vi "Host-Scannig-Probe-Microscope-Controller-2010-06-05-RFR-1a-version-for-MCL-drift-trial-fm-NanoH50 D082914.vi"() -> ()   [LabVIEW 2012]
uses:
  <vilib>/FPGAPlugInAG/PCI-7831R/niLvFpga_Open_PCI-7831R.vi
  <vilib>/Utility/error.llb/Error Cluster From Error Code.vi
  <vilib>/rvi/errors/niLvFpgaAdjustHostInterfaceError.vi
  <vilib>/FPGAPlugInAG/PCI-7831R/niLvFpga_Close_PCI-7831R.vi
  <vilib>/FPGAPlugInAG/PCI-7831R/niLvFpga_Run_PCI-7831R.vi
  <vilib>/Utility/file.llb/Write To Spreadsheet File (I64).vi
  <vilib>/rvi/interface/nirviOpenFPGA/nirviOpenFPGA.xnode
  Documents/FPGA-project-apporach-retraction/FPGA Bitfiles/Apporach-Retract_FPGATarget_Scannig-Probe-Mi_0gtNGMjHE5o.lvbitx
  Scannig-Probe-Microscope-Controller-2010-03-08-RFR-1a-version-for-MCL-drift-trial-fm-multiple-channels-nanoh50.vi
  <vilib>/rvi/interface/nirviMethod/nirviMethod.xnode
  <vilib>/rvi/interface/nirviReadWriteControl/nirviReadWriteControl.xnode
  <vilib>/rvi/interface/nirviCloseFPGA/nirviCloseFPGA.xnode
  <vilib>/rvi/errors/niLvFpgaMergeErrorWithErrorCode.vi
  NiFpgaLv.dll
  <vilib>/FPGAPlugInAG/PCI-7831R/niLvFpga_ReadFifo_PCI-7831R.vi
panel:
  out "fpga y images":i32
  out "hi(x)":u16[](array[numeric])=[65532, 21, 65429, 46, 65369, 15, 65513, 65465, 46, 65357, 35, 65457, 65513, 26, 65398, 44, 65387, 9, 4, 65453, 44, 65356, 26, 65480, 65489, 30, 65375, 36, 65416, 3, 18, 65446, 48, 65359, 19, 65504, 65469, 44, 65360, 34, 65444, 65519, 25, 65408, 47, 65382, 13, 65532, 65458, 44, 65353, 30, 65471, 65495, 30, 65383, 42, 65407, 6, 13, 65452, 48, 65368, 21, 65495, 65473, 39, 65364, 37, 65438, 65528, 23, 65411, 46, 65377, 13, 65524, 65460, 44, 65353, 32, 65464, 65502, 26, 65391, 43, 65397, 6, 9, 65450, 46, 65362, 25, 65486, 65480, 27, 65365, 42, 65424, 65533, 23, 65423, 47, 65371, 15, 65514, 65464, 42, 65355, 31, 65456, 65506, 26, 65394, 45, 65389, 9, 6, 65453, 47, 65354, 25, 65478, 65484, 28, 65374, 34, 65417, 0, 21, 65435, 47, 65359, 18, 65507, 65468, 46, 65356, 34, 65448, 65517, 26, 65405, 44, 65386, 11, 65535, 65457, 46, 65355, 28, 65476, 65492, 29, 65377, 42, 65410, 3, 18, 65454, 48, 65363, 20, 65501, 65473, 39, 65359, 36, 65438, 65524, 24, 65410, 46, 65380, 13, 65531, 65460, 46, 65355, 31, 65467, 65497, 28, 65384, 42, 65402, 7, 13, 65449, 46, 65368, 23, 65490, 65477, 35, 65366, 40, 65432, 65529, 22, 65417, 47, 65374, 14, 65519, 65464, 42, 65354, 31, 65460, 65501, 28, 65393, 46, 65395, 9, 8, 65453, 48, 65356, 26, 65483, 65482, 21, 65368, 39, 65423, 65533, 23, 65429, 48, 65367, 17, 65510, 65466, 46, 65357, 33, 65451, 65510, 23, 65400, 43, 65389, 10, 2, 65455, 47, 65353, 26, 65476, 65490, 28, 65378, 35, 65413]
  out "Y line":i32=81
  out "Time per step (us) /X axis sub pixels":u32=1220
  in  "X axis pixels":u16=512
  in  "Lines per second":dbl=0.2 min=1e-05 max=50.0
  in  "Time per step/ Y axis sub pixels (usec)":u32=1200
  in  "X Size (um)":dbl=10.0
  in  "X Total Range (um)":dbl=80.0
  in  "Y Size (um)":dbl=10.0
  in  "Y Total Range (um)":dbl=80.0
  in  "Y axis pixels":u16=512
  in  "Timeout FIFO":i32=-1
  in  "x initial":i16=-32760
  in  "y initial":i16=-32710
  out "X axis steps per pixel":u16=8
  in  "Number of images":u32=10000
  out "Y axis steps per pixel":u16=8
  out "Pixels for one image":i32=524288
  in  "Internal Setpoint":i16=7166
  in  "I scale":i8=-8
  in  "P scale":i8
  in  "Setpoint Control":bool=TRUE
  in  "PID gains (x 2^8)":T1={"proportional gain (Kc)"=1, "integral gain (Kc*Ts/Ti)"=11, "derivative gain (Kc*Td/Ts)"=0}
  in  "Forth/Back X axis":bool
  in  "Forth/Back Y axis":bool
  in  "Feedback loop time(uSec)":u8
  in  "Stop Feedback":bool=TRUE
  in  "Scanning On/Off":bool
  in  "control for drift correction":u32=512000
  out "Steps Per Feedback region":u16=642
  in  "Number of Feedback Regions":u32=102
  in  "upper limit regions":i16=99
  out "line shift":i32=-1
  out "line in matrix":i32=80
  out "Y Output Value":i16=-32054
  out "image indicator":i32
  out "Bottom Sensor Magnitude Image":i16[][](graph)
  out "Trace Bottom Sensor Magnitude":i16[][](graph)=[[41, 50, 79, 100, 124, 92, 130, 194, 155, 119, 90, 52, 169, 196, 52, 81, 107, 97, 38, 169, 150, 28, 89, 84, 18, 25, 51, 184, 150, 110, 155, 167, 122, 228, 203, 75, 201, 101, 167, 149, 80, 89, 32, 120, 164, 110, 260, 104, 77, 34, 69, 125, 141, 131, 177, 43, 257, 242, 80, 65, 98, 218, 145, 115, 125, 34, 174, 80, 78, 182, 63, 67, -5, 186, 59, 112, 169, 133, 153, 205, 220, 231, 179, -6, 137, 135, 104, 121, 121, 4, 32, 127, 149, 22, 158, 160, 147, 32, -108, 132, 241, 134, 185, 77, 233, 197, 268, 26, 211, 313, 123, 22, 29, 158, 139, 153, 155, 139, 230, 147, 12, 119, 36, 53, 226, 114, 18, 89, 167, 226, 89, 114, 39, 114, 146, 82, 117, 210, 120, 130, 89, 242, 66, 50, 63, 89, 215, 93, 202, 62, 217, 101, 72, 108, 107, 230, 75, 124, 178, 145, 151, 112, 161, 160, 128, 42, 134, 109, -52, 159, 142, 126, 57, 230, 7, 151, 27, 129, 87, 148, 174, 142, 215, 110, 88, 45, 88, 43, 146, 227, 61, 262, 158, 118, 154, 142, 53, 207, 196, 101, 8, 132, 58, 74, 95, 69, 131, 226, 161, 109, 62, 212, 3, 20, 207, 111, 193, 73, 242, 114, -14, 170, 48, 4, 172, 90, 96, 287, -18, 98, 30, 147, 228, 145, 109, 136, 208, 182, 156, 163, 119, 305, 172, 81, 230, 199, 73, 148, 62, 266, 63, 82, 17, 132, 77, 305, 38, 6, 50, 233, -5, 164, 215, 85, 188, 159, 89, 148, 139, 127, 68, 84, 64, 238, 9, 122, 235, 77, 234, 71, 177, 104, 123, 214, 172, 130, 85, 121, 161, 251, 152, 66, 171, 109, 58, 62, 176, 92, 94, 126, 180, 228, 42, 122, 190, 41, 40, 153, 163, 53, 217, 123, 118, 264, 64, 154, 144, 148, 118, 109, 101, 11, 203, 147, 25, 144, 81, 112, 73, 203, -57, 181, 123, 193, 104, 135, 17, 56, 129, 13, 50, 44, 147, 27, 109, 142, 56, 62, 32, 58, 140, 83, 227, 195, 134, 215, 50, 203, 102, 86, 208, 209, 139, 108, -58, 11, 72, 101, 138, 63, 137, 68, -11, 42, 1, 134, 216, 138, 188, 215, 64, 8, 187, 93, 120, 168, 70, 177, 149, 89, 212, 163, 106, 81, 168, 123, 21, 162, 185, 136, 154, 242, 215, 20, 57, 91, 132, 166, 53, 82, 128, 161, 135, 157, 35, 205, 194, 101, 103, 69, 37, 127, 227, 263, 80, 125, 186, 204, 287, 183, 120, 125, 86, 101, 166, 236, 53, 84, 129, 184, 176, 178, 174, 93, 163, 270, 115, 249, 64, 138, 89, 95, 118, 130, 80, 148, 289, 86, 28, 138, 90, -9, 254, -56, 149, 109, 109, 200, 191, 115, 157, 157, 104, 51, 114, 153, 143, 244, 163, 134, 201, 38, 224, 75, 191, 52, 102, 58, 133, 48, 107, 72, 153, 156, 112, 192, 141, 256, 86, 107, 219, 83, 42, 109, 20, 138, 149, 132, 110, 40, 88, 109], [237, 108, 67, 210, -4, 118, 207, 137, 134, 154, 46, 91, 85, 154, 186, 70, 135, 69, 110, 172, 208, 152, 193, 103, 111, 178, 97, 183, 209, 67, 119, 163, 212, 109, 20, 163, 7, 190, 70, -17, 66, 151, 91, 93, 120, 178, 145, 129, 219, 78, 111, 87, 86, 155, 94, 93, 54, 109, 153, 159, 144, 111, 80, 104, 64, 79, 156, 141, 82, 143, -2, 71, 150, 232, 121, 3, 232, 88, 36, 47, 193, 81, 106, 144, 106, 72, 124, 213, 165, 117, 153, 159, 162, 120, 325, 90, 117, 87, 87, 133, -6, 137, 137, 167, 112, 108, 23, 81, 70, 158, 146, 83, 137, -24, 100, 138, 131, 102, 95, -69, 87, 125, 183, 60, 33, 56, 167, 231, 74, 171, 165, 206, 70, 64, 21, 211, 148, 52, 153, 198, 80, 101, 140, 147, 69, 206, 166, 42, -16, 164, 160, 116, 64, 72, 121, 99, 128, 140, 85, 82, 170, 265, 192, 175, -2, 181, 123, 92, 101, 162, 136, 82, 246, 86, 9, 62, 126, 144, 57, 152, 167, 16, 94, 105, 137, 26, 186, -33, 135, 104, 136, 183, 150, 33, 124, 56, 87, 26, 196, 107, 136, 185, 156, 173, 4, 134, 42, 232, 81, 219, 55, 3, 133, -19, 83, 286, 83, 75, 38, 219, 116, 114, 189, 196, 119, 84, 196, 88, 111, 169, -24, 139, 173, 87, 230, 56, 182, 110, 155, 154, 113, 148, 155, 141, 61, 133, 88, 163, 144, 110, 241, 108, 112, 64, 194, -2, 89, 191, 94, -9, -30, 82, 203, 109, 142, 5, 71, 135, 185, 118, 98, 106, 40, 112, 120, 41, 124, 172, 67, 21, 123, 242, 256, 164, 121, 156, 87, 39, 174, 48, 107, 190, 31, 272, 98, 79, 133, -45, 80, 38, 143, 69, 151, 188, 149, 122, 97, 95, 112, -25, 208, 87, 197, 218, 72, 141, 9, 66, 35, 140, 51, 51, 196, 189, 150, 61, 183, 227, 139, -11, 150, 161, 5, 64, 174, 43, 230, 131, 25, 170, 96, 226, 93, 184, 69, 118, 240, 96, 215, 39, 169, 40, 252, 140, 135, 133, 284, 192, 100, 110, 99, 114, 56, 50, 83, 63, -8, 158, 66, -4, 168, 79, 233, 28, 35, 199, 110, 116, 141, 191, 77, 45, 123, 158, 17, 150, 162, 164, 84, 72, 90, 91, 88, 98, 195, 98, 178, 169, 217, 196, 27, 220, 92, 129, 165, 111, 150, 74, 93, 203, 103, 142, 132, 128, 13, 101, 143, 178, 72, -13, 185, -42, 134, 78, 157, 114, 112, 77, 59, 172, 105, 224, 79, 73, -16, 46, 116, 163, 134, 120, 123, 133, 81, -8, 214, 227, 117, 39, 225, 198, 12, 55, 93, 228, 90, 61, 106, 20, 57, 53, 144, 64, 67, 213, 8, 97, 232, 133, 119, 224, 70, 158, 228, 218, 154, 189, 141, 139, 183, 73, 70, 46, 202, 41, 236, 112, 94, 95, 47, 55, 45, 201, -8, 114, 136, 46, 21, 42, 137, 107, 47, 253, 20, 186, 118, 177, 163, 130, 105, 59, 214, 186]]
  out "TF Magnitude Image":i16[][](graph)
  out "Trace TF Magnitud":i16[][](graph)=[[-1059, -1061, -1058, -1061, -1059, -1062, -1059, -1060, -1061, -1060, -1059, -1061, -1060, -1059, -1062, -1061, -1059, -1061, -1061, -1059, -1060, -1060, -1063, -1061, -1062, -1062, -1059, -1056, -1062, -1058, -1060, -1059, -1061, -1060, -1059, -1061, -1058, -1061, -1060, -1062, -1061, -1059, -1060, -1060, -1061, -1059, -1057, -1060, -1061, -1060, -1059, -1060, -1060, -1060, -1060, -1060, -1058, -1060, -1058, -1061, -1060, -1058, -1060, -1061, -1059, -1059, -1060, -1059, -1062, -1059, -1061, -1060, -1061, -1060, -1060, -1060, -1060, -1059, -1061, -1059, -1059, -1057, -1063, -1058, -1061, -1061, -1061, -1061, -1059, -1060, -1061, -1059, -1062, -1059, -1059, -1060, -1059, -1060, -1061, -1060, -1060, -1059, -1060, -1060, -1058, -1057, -1062, -1060, -1059, -1059, -1058, -1060, -1061, -1060, -1059, -1059, -1062, -1059, -1060, -1060, -1058, -1061, -1062, -1060, -1058, -1062, -1053, -1061, -1058, -1060, -1060, -1059, -1062, -1060, -1061, -1056, -1059, -1058, -1058, -1059, -1059, -1062, -1061, -1058, -1060, -1060, -1062, -1061, -1061, -1061, -1061, -1059, -1059, -1058, -1060, -1058, -1061, -1060, -1062, -1060, -1061, -1058, -1057, -1060, -1061, -1062, -1060, -1061, -1060, -1060, -1060, -1058, -1060, -1059, -1060, -1060, -1062, -1059, -1058, -1060, -1060, -1063, -1061, -1058, -1061, -1059, -1061, -1061, -1061, -1057, -1059, -1058, -1061, -1061, -1061, -1061, -1062, -1061, -1061, -1059, -1059, -1058, -1061, -1061, -1062, -1059, -1058, -1061, -1060, -1061, -1059, -1058, -1060, -1060, -1058, -1060, -1059, -1062, -1060, -1061, -1061, -1060, -1062, -1061, -1059, -1062, -1062, -1059, -1062, -1061, -1061, -1060, -1060, -1060, -1059, -1059, -1059, -1062, -1059, -1059, -1060, -1060, -1061, -1059, -1059, -1060, -1061, -1059, -1060, -1059, -1059, -1060, -1060, -1060, -1062, -1059, -1060, -1062, -1059, -1057, -1061, -1059, -1057, -1060, -1057, -1058, -1059, -1058, -1060, -1059, -1059, -1060, -1059, -1059, -1060, -1062, -1055, -1060, -1059, -1058, -1059, -1059, -1059, -1061, -1060, -1059, -1057, -1059, -1059, -1061, -1060, -1058, -1057, -1061, -1062, -1060, -1060, -1058, -1061, -1059, -1058, -1058, -1061, -1061, -1061, -1060, -1062, -1061, -1060, -1059, -1058, -1062, -1061, -1058, -1061, -1058, -1059, -1059, -1061, -1062, -1061, -1061, -1060, -1061, -1052, -1060, -1062, -1060, -1061, -1059, -1060, -1060, -1061, -1059, -1061, -1061, -1061, -1062, -1061, -1062, -1061, -1061, -1060, -1060, -1060, -1061, -1059, -1063, -1062, -1061, -1062, -1062, -1060, -1062, -1060, -1060, -1060, -1062, -1058, -1059, -1060, -1057, -1059, -1060, -1064, -1061, -1059, -1059, -1059, -1061, -1059, -1059, -1061, -1058, -1061, -1059, -1058, -1058, -1060, -1061, -1061, -1060, -1058, -1060, -1060, -1060, -1062, -1061, -1059, -1059, -1059, -1059, -1059, -1059, -1059, -1060, -1061, -1059, -1058, -1058, -1061, -1057, -1057, -1060, -1061, -1058, -1061, -1061, -1055, -1059, -1060, -1059, -1061, -1060, -1059, -1057, -1059, -1062, -1060, -1061, -1061, -1058, -1061, -1060, -1061, -1057, -1061, -1059, -1061, -1059, -1056, -1059, -1060, -1059, -1062, -1059, -1059, -1059, -1059, -1057, -1058, -1060, -1060, -1060, -1057, -1057, -1058, -1061, -1062, -1060, -1059, -1060, -1060, -1059, -1060, -1061, -1060, -1059, -1061, -1059, -1058, -1061, -1059, -1058, -1061, -1060, -1060, -1057, -1060, -1062, -1059, -1059, -1058, -1062, -1058, -1062, -1059, -1060, -1061, -1058, -1060, -1061, -1057, -1059, -1062, -1061, -1059, -1061, -1059, -1060, -1063, -1059, -1059, -1060, -1063, -1061, -1059, -1059, -1059, -1059, -1058, -1063, -1060, -1060, -1061, -1059, -1062, -1063, -1060, -1058, -1059, -1058], [-1057, -1058, -1060, -1059, -1061, -1060, -1059, -1061, -1057, -1060, -1062, -1060, -1060, -1060, -1057, -1060, -1057, -1060, -1059, -1060, -1060, -1061, -1060, -1059, -1060, -1059, -1057, -1062, -1058, -1062, -1056, -1059, -1059, -1061, -1058, -1061, -1058, -1059, -1061, -1059, -1061, -1059, -1059, -1059, -1061, -1058, -1059, -1057, -1058, -1060, -1062, -1060, -1058, -1060, -1061, -1060, -1059, -1057, -1059, -1060, -1059, -1058, -1059, -1064, -1061, -1061, -1059, -1061, -1059, -1060, -1061, -1058, -1060, -1057, -1060, -1060, -1058, -1059, -1059, -1059, -1060, -1059, -1060, -1062, -1061, -1059, -1059, -1059, -1059, -1060, -1061, -1058, -1060, -1059, -1057, -1059, -1060, -1060, -1062, -1061, -1060, -1058, -1063, -1058, -1060, -1062, -1061, -1058, -1060, -1060, -1059, -1061, -1060, -1061, -1059, -1060, -1056, -1059, -1060, -1060, -1059, -1060, -1060, -1060, -1060, -1059, -1060, -1059, -1060, -1060, -1060, -1059, -1061, -1062, -1060, -1059, -1059, -1062, -1058, -1057, -1062, -1059, -1060, -1059, -1058, -1058, -1057, -1061, -1060, -1061, -1058, -1061, -1059, -1059, -1060, -1060, -1060, -1057, -1058, -1060, -1062, -1057, -1057, -1059, -1061, -1060, -1060, -1059, -1060, -1060, -1058, -1060, -1061, -1060, -1060, -1059, -1062, -1060, -1060, -1062, -1060, -1060, -1059, -1062, -1059, -1061, -1059, -1062, -1059, -1059, -1059, -1060, -1062, -1061, -1061, -1060, -1061, -1062, -1058, -1064, -1061, -1059, -1060, -1060, -1063, -1061, -1060, -1057, -1062, -1062, -1061, -1060, -1062, -1060, -1062, -1057, -1061, -1061, -1058, -1061, -1061, -1059, -1061, -1057, -1060, -1060, -1060, -1060, -1060, -1060, -1061, -1060, -1060, -1060, -1060, -1061, -1059, -1059, -1060, -1056, -1061, -1060, -1057, -1059, -1061, -1060, -1062, -1059, -1056, -1056, -1061, -1060, -1057, -1059, -1060, -1058, -1059, -1060, -1059, -1060, -1060, -1060, -1061, -1060, -1060, -1057, -1058, -1059, -1057, -1061, -1058, -1062, -1060, -1057, -1061, -1061, -1060, -1061, -1059, -1062, -1057, -1061, -1058, -1061, -1058, -1057, -1060, -1060, -1059, -1060, -1060, -1057, -1062, -1059, -1060, -1061, -1058, -1059, -1060, -1061, -1059, -1060, -1058, -1059, -1060, -1059, -1060, -1059, -1061, -1060, -1058, -1060, -1061, -1060, -1058, -1059, -1060, -1060, -1060, -1060, -1061, -1061, -1062, -1058, -1061, -1061, -1060, -1059, -1059, -1059, -1059, -1060, -1061, -1059, -1059, -1059, -1059, -1061, -1060, -1060, -1060, -1058, -1061, -1060, -1056, -1060, -1058, -1060, -1061, -1060, -1061, -1063, -1058, -1057, -1059, -1060, -1062, -1062, -1061, -1061, -1060, -1060, -1061, -1060, -1061, -1060, -1063, -1058, -1059, -1058, -1060, -1058, -1055, -1061, -1061, -1059, -1058, -1060, -1061, -1061, -1059, -1062, -1060, -1060, -1061, -1060, -1061, -1060, -1061, -1059, -1060, -1059, -1058, -1060, -1059, -1062, -1061, -1058, -1061, -1060, -1062, -1059, -1059, -1060, -1061, -1062, -1058, -1061, -1060, -1060, -1060, -1059, -1060, -1063, -1059, -1060, -1061, -1060, -1062, -1061, -1061, -1062, -1059, -1057, -1062, -1065, -1059, -1061, -1058, -1061, -1061, -1059, -1060, -1058, -1060, -1061, -1060, -1059, -1060, -1059, -1063, -1062, -1059, -1064, -1060, -1061, -1061, -1062, -1058, -1060, -1061, -1060, -1059, -1059, -1061, -1057, -1059, -1060, -1058, -1060, -1060, -1062, -1060, -1059, -1061, -1061, -1059, -1060, -1060, -1059, -1060, -1057, -1060, -1057, -1060, -1060, -1060, -1059, -1059, -1061, -1060, -1060, -1059, -1060, -1058, -1060, -1060, -1063, -1063, -1061, -1060, -1059, -1061, -1058, -1060, -1061, -1059, -1059, -1060, -1063, -1063, -1058, -1061, -1060, -1057, -1061, -1060, -1059, -1061, -1058, -1062, -1058]]
  out "Trace AI5 array":i16[][](array[numeric])=[[41, 50, 79, 100, 124, 92, 130, 194, 155, 119, 90, 52, 169, 196, 52, 81, 107, 97, 38, 169, 150, 28, 89, 84, 18, 25, 51, 184, 150, 110, 155, 167, 122, 228, 203, 75, 201, 101, 167, 149, 80, 89, 32, 120, 164, 110, 260, 104, 77, 34, 69, 125, 141, 131, 177, 43, 257, 242, 80, 65, 98, 218, 145, 115, 125, 34, 174, 80, 78, 182, 63, 67, -5, 186, 59, 112, 169, 133, 153, 205, 220, 231, 179, -6, 137, 135, 104, 121, 121, 4, 32, 127, 149, 22, 158, 160, 147, 32, -108, 132, 241, 134, 185, 77, 233, 197, 268, 26, 211, 313, 123, 22, 29, 158, 139, 153, 155, 139, 230, 147, 12, 119, 36, 53, 226, 114, 18, 89, 167, 226, 89, 114, 39, 114, 146, 82, 117, 210, 120, 130, 89, 242, 66, 50, 63, 89, 215, 93, 202, 62, 217, 101, 72, 108, 107, 230, 75, 124, 178, 145, 151, 112, 161, 160, 128, 42, 134, 109, -52, 159, 142, 126, 57, 230, 7, 151, 27, 129, 87, 148, 174, 142, 215, 110, 88, 45, 88, 43, 146, 227, 61, 262, 158, 118, 154, 142, 53, 207, 196, 101, 8, 132, 58, 74, 95, 69, 131, 226, 161, 109, 62, 212, 3, 20, 207, 111, 193, 73, 242, 114, -14, 170, 48, 4, 172, 90, 96, 287, -18, 98, 30, 147, 228, 145, 109, 136, 208, 182, 156, 163, 119, 305, 172, 81, 230, 199, 73, 148, 62, 266, 63, 82, 17, 132, 77, 305, 38, 6, 50, 233, -5, 164, 215, 85, 188, 159, 89, 148, 139, 127, 68, 84, 64, 238, 9, 122, 235, 77, 234, 71, 177, 104, 123, 214, 172, 130, 85, 121, 161, 251, 152, 66, 171, 109, 58, 62, 176, 92, 94, 126, 180, 228, 42, 122, 190, 41, 40, 153, 163, 53, 217, 123, 118, 264, 64, 154, 144, 148, 118, 109, 101, 11, 203, 147, 25, 144, 81, 112, 73, 203, -57, 181, 123, 193, 104, 135, 17, 56, 129, 13, 50, 44, 147, 27, 109, 142, 56, 62, 32, 58, 140, 83, 227, 195, 134, 215, 50, 203, 102, 86, 208, 209, 139, 108, -58, 11, 72, 101, 138, 63, 137, 68, -11, 42, 1, 134, 216, 138, 188, 215, 64, 8, 187, 93, 120, 168, 70, 177, 149, 89, 212, 163, 106, 81, 168, 123, 21, 162, 185, 136, 154, 242, 215, 20, 57, 91, 132, 166, 53, 82, 128, 161, 135, 157, 35, 205, 194, 101, 103, 69, 37, 127, 227, 263, 80, 125, 186, 204, 287, 183, 120, 125, 86, 101, 166, 236, 53, 84, 129, 184, 176, 178, 174, 93, 163, 270, 115, 249, 64, 138, 89, 95, 118, 130, 80, 148, 289, 86, 28, 138, 90, -9, 254, -56, 149, 109, 109, 200, 191, 115, 157, 157, 104, 51, 114, 153, 143, 244, 163, 134, 201, 38, 224, 75, 191, 52, 102, 58, 133, 48, 107, 72, 153, 156, 112, 192, 141, 256, 86, 107, 219, 83, 42, 109, 20, 138, 149, 132, 110, 40, 88, 109], [237, 108, 67, 210, -4, 118, 207, 137, 134, 154, 46, 91, 85, 154, 186, 70, 135, 69, 110, 172, 208, 152, 193, 103, 111, 178, 97, 183, 209, 67, 119, 163, 212, 109, 20, 163, 7, 190, 70, -17, 66, 151, 91, 93, 120, 178, 145, 129, 219, 78, 111, 87, 86, 155, 94, 93, 54, 109, 153, 159, 144, 111, 80, 104, 64, 79, 156, 141, 82, 143, -2, 71, 150, 232, 121, 3, 232, 88, 36, 47, 193, 81, 106, 144, 106, 72, 124, 213, 165, 117, 153, 159, 162, 120, 325, 90, 117, 87, 87, 133, -6, 137, 137, 167, 112, 108, 23, 81, 70, 158, 146, 83, 137, -24, 100, 138, 131, 102, 95, -69, 87, 125, 183, 60, 33, 56, 167, 231, 74, 171, 165, 206, 70, 64, 21, 211, 148, 52, 153, 198, 80, 101, 140, 147, 69, 206, 166, 42, -16, 164, 160, 116, 64, 72, 121, 99, 128, 140, 85, 82, 170, 265, 192, 175, -2, 181, 123, 92, 101, 162, 136, 82, 246, 86, 9, 62, 126, 144, 57, 152, 167, 16, 94, 105, 137, 26, 186, -33, 135, 104, 136, 183, 150, 33, 124, 56, 87, 26, 196, 107, 136, 185, 156, 173, 4, 134, 42, 232, 81, 219, 55, 3, 133, -19, 83, 286, 83, 75, 38, 219, 116, 114, 189, 196, 119, 84, 196, 88, 111, 169, -24, 139, 173, 87, 230, 56, 182, 110, 155, 154, 113, 148, 155, 141, 61, 133, 88, 163, 144, 110, 241, 108, 112, 64, 194, -2, 89, 191, 94, -9, -30, 82, 203, 109, 142, 5, 71, 135, 185, 118, 98, 106, 40, 112, 120, 41, 124, 172, 67, 21, 123, 242, 256, 164, 121, 156, 87, 39, 174, 48, 107, 190, 31, 272, 98, 79, 133, -45, 80, 38, 143, 69, 151, 188, 149, 122, 97, 95, 112, -25, 208, 87, 197, 218, 72, 141, 9, 66, 35, 140, 51, 51, 196, 189, 150, 61, 183, 227, 139, -11, 150, 161, 5, 64, 174, 43, 230, 131, 25, 170, 96, 226, 93, 184, 69, 118, 240, 96, 215, 39, 169, 40, 252, 140, 135, 133, 284, 192, 100, 110, 99, 114, 56, 50, 83, 63, -8, 158, 66, -4, 168, 79, 233, 28, 35, 199, 110, 116, 141, 191, 77, 45, 123, 158, 17, 150, 162, 164, 84, 72, 90, 91, 88, 98, 195, 98, 178, 169, 217, 196, 27, 220, 92, 129, 165, 111, 150, 74, 93, 203, 103, 142, 132, 128, 13, 101, 143, 178, 72, -13, 185, -42, 134, 78, 157, 114, 112, 77, 59, 172, 105, 224, 79, 73, -16, 46, 116, 163, 134, 120, 123, 133, 81, -8, 214, 227, 117, 39, 225, 198, 12, 55, 93, 228, 90, 61, 106, 20, 57, 53, 144, 64, 67, 213, 8, 97, 232, 133, 119, 224, 70, 158, 228, 218, 154, 189, 141, 139, 183, 73, 70, 46, 202, 41, 236, 112, 94, 95, 47, 55, 45, 201, -8, 114, 136, 46, 21, 42, 137, 107, 47, 253, 20, 186, 118, 177, 163, 130, 105, 59, 214, 186]]
  out "Trace AI5 temp":i16[](array[numeric])=[54, 151, 139, 139, 176, 3, 95, 63, 94, 117, 40, 198, 140, 226, 89, 129, 122, 115, 125, 198, 114, 199, 172, -33, 154, 113, 26, 61, 166, 124, 137, 48, 150, 145, 106, 30, 92, 95, -27, 280, 207, 128, 67, 20, 85, 155, 27, 159, 250, 127, 137, 135, 76, 149, 265, 148, 181, 6, -14, 177, 118, 132, 185, 76, 84, 23, 220, 166, 117, 73, 60, 94, 218, 108, 122, 76, 97, 57, 101, 133, 106, 52, 213, 117, 91, 203, 72, 19, 167, 107, 152, 237, 120, 175, 209, 12, 220, 53, 237, 121, 136, -82, 173, 57, 39, 127, 94, 149, 176, 184, 117, 40, 44, 118, 191, 125, 91, 45, -32, 227, 141, 182, 112, 95, 7, 45, 178, 201, 208, 181, 85, 109, 135, 49, 188, 187, 60, 54, 100, 116, 115, 130, 125, 189, 102, -61, 133, 159, 154, 107, 181, 239, 50, 117, 184, 67, 161, 149, 63, 177, 111, 121, 81, 101, 42, 277, 121, 98, 56, 128, 125, 196, 139, 155, 168, 197, 141, 114, 143, 97, 106, 42, 231, 85, 222, 139, 86, 118, 127, 86, -37, 62, 224, 9, 10, 132, 133, 213, 76, 73, 181, 46, 200, 77, 145, 208, 111, 82, 35, 123, 22, 72, 142, 99, 75, 217, 190, 189, 215, 221, 136, 138, 196, 57, 43, 145, 163, 147, 114, 97, 159, 246, 181, -17, 117, 156, 128, 86, 142, 232, 14, 218, 68, 178, 79, 142, 43, 152, 172, 104, 54, 95, 107, 163, 188, 88, 87, 160, 97, 101, 88, 34, 26, 171, 43, 45, 91, 36, 213, -103, 272, 152, 177, 143, 38, 124, 42, 162, 52, 47, 155, 131, 135, 52, 148, 152, 163, 103, 126, 185, 184, 232, 99, 47, 231, 96, 120, 194, 43, 82, 189, 262, 102, 83, 52, 156, 24, 126, 77, 195, 24, 119, 114, 134, 280, 259, 118, 39, 118, 115, 136, 190, 147, 129, 58, 132, 29, 127, 219, 59, 58, 87, 213, 126, 221, 65, 202, 54, 98, 279, -80, 98, 110, 108, 168, 79, 131, 132, -31, 124, 155, 62, 314, 26, 205, 111, -37, 15, 158, 83, 129, 13, 153, 198, 71, 85, -13, 63, 242, 108, 81, 144, 20, 175, 80, 46, 88, 207, 136, 43, 205, -17, 211, 206, 134, 90, 139, 61, 71, 170, 201, 39, 12, 295, 119, 160, 132, 14, 170, 19, 127, 78, 157, 141, 148, 127, 173, 11, 66, 178, 12, 180, 138, 231, 46, 214, 15, 146, -20, -11, 185, 91, 88, 15, 51, 101, -29, 63, 192, 120, 179, 66, 48, 85, 45, 214, 139, 24, 163, 196, 142, 88, 169, 192, 36, 141, 124, 121, 189, 139, 4, 57, 86, 56, 170, 104, 66, 201, 121, 79, 188, 126, 96, 168, 110, 251, 86, 82, 99, 131, 149, 105, 111, 79, 194, 153, 129, 65, 120, 226, 199, 103, 28, 197, 239, 277, 13, 222, 116, 74, 258, 59, 118, 336, 126, 140, 316, 51, 107, 86, 48, 36, 171, 133, 97, 114, 131, 151, 169, 39, 189, 135]
  out "Trace AI6  array":i16[][](array[numeric])=[[-1059, -1061, -1058, -1061, -1059, -1062, -1059, -1060, -1061, -1060, -1059, -1061, -1060, -1059, -1062, -1061, -1059, -1061, -1061, -1059, -1060, -1060, -1063, -1061, -1062, -1062, -1059, -1056, -1062, -1058, -1060, -1059, -1061, -1060, -1059, -1061, -1058, -1061, -1060, -1062, -1061, -1059, -1060, -1060, -1061, -1059, -1057, -1060, -1061, -1060, -1059, -1060, -1060, -1060, -1060, -1060, -1058, -1060, -1058, -1061, -1060, -1058, -1060, -1061, -1059, -1059, -1060, -1059, -1062, -1059, -1061, -1060, -1061, -1060, -1060, -1060, -1060, -1059, -1061, -1059, -1059, -1057, -1063, -1058, -1061, -1061, -1061, -1061, -1059, -1060, -1061, -1059, -1062, -1059, -1059, -1060, -1059, -1060, -1061, -1060, -1060, -1059, -1060, -1060, -1058, -1057, -1062, -1060, -1059, -1059, -1058, -1060, -1061, -1060, -1059, -1059, -1062, -1059, -1060, -1060, -1058, -1061, -1062, -1060, -1058, -1062, -1053, -1061, -1058, -1060, -1060, -1059, -1062, -1060, -1061, -1056, -1059, -1058, -1058, -1059, -1059, -1062, -1061, -1058, -1060, -1060, -1062, -1061, -1061, -1061, -1061, -1059, -1059, -1058, -1060, -1058, -1061, -1060, -1062, -1060, -1061, -1058, -1057, -1060, -1061, -1062, -1060, -1061, -1060, -1060, -1060, -1058, -1060, -1059, -1060, -1060, -1062, -1059, -1058, -1060, -1060, -1063, -1061, -1058, -1061, -1059, -1061, -1061, -1061, -1057, -1059, -1058, -1061, -1061, -1061, -1061, -1062, -1061, -1061, -1059, -1059, -1058, -1061, -1061, -1062, -1059, -1058, -1061, -1060, -1061, -1059, -1058, -1060, -1060, -1058, -1060, -1059, -1062, -1060, -1061, -1061, -1060, -1062, -1061, -1059, -1062, -1062, -1059, -1062, -1061, -1061, -1060, -1060, -1060, -1059, -1059, -1059, -1062, -1059, -1059, -1060, -1060, -1061, -1059, -1059, -1060, -1061, -1059, -1060, -1059, -1059, -1060, -1060, -1060, -1062, -1059, -1060, -1062, -1059, -1057, -1061, -1059, -1057, -1060, -1057, -1058, -1059, -1058, -1060, -1059, -1059, -1060, -1059, -1059, -1060, -1062, -1055, -1060, -1059, -1058, -1059, -1059, -1059, -1061, -1060, -1059, -1057, -1059, -1059, -1061, -1060, -1058, -1057, -1061, -1062, -1060, -1060, -1058, -1061, -1059, -1058, -1058, -1061, -1061, -1061, -1060, -1062, -1061, -1060, -1059, -1058, -1062, -1061, -1058, -1061, -1058, -1059, -1059, -1061, -1062, -1061, -1061, -1060, -1061, -1052, -1060, -1062, -1060, -1061, -1059, -1060, -1060, -1061, -1059, -1061, -1061, -1061, -1062, -1061, -1062, -1061, -1061, -1060, -1060, -1060, -1061, -1059, -1063, -1062, -1061, -1062, -1062, -1060, -1062, -1060, -1060, -1060, -1062, -1058, -1059, -1060, -1057, -1059, -1060, -1064, -1061, -1059, -1059, -1059, -1061, -1059, -1059, -1061, -1058, -1061, -1059, -1058, -1058, -1060, -1061, -1061, -1060, -1058, -1060, -1060, -1060, -1062, -1061, -1059, -1059, -1059, -1059, -1059, -1059, -1059, -1060, -1061, -1059, -1058, -1058, -1061, -1057, -1057, -1060, -1061, -1058, -1061, -1061, -1055, -1059, -1060, -1059, -1061, -1060, -1059, -1057, -1059, -1062, -1060, -1061, -1061, -1058, -1061, -1060, -1061, -1057, -1061, -1059, -1061, -1059, -1056, -1059, -1060, -1059, -1062, -1059, -1059, -1059, -1059, -1057, -1058, -1060, -1060, -1060, -1057, -1057, -1058, -1061, -1062, -1060, -1059, -1060, -1060, -1059, -1060, -1061, -1060, -1059, -1061, -1059, -1058, -1061, -1059, -1058, -1061, -1060, -1060, -1057, -1060, -1062, -1059, -1059, -1058, -1062, -1058, -1062, -1059, -1060, -1061, -1058, -1060, -1061, -1057, -1059, -1062, -1061, -1059, -1061, -1059, -1060, -1063, -1059, -1059, -1060, -1063, -1061, -1059, -1059, -1059, -1059, -1058, -1063, -1060, -1060, -1061, -1059, -1062, -1063, -1060, -1058, -1059, -1058], [-1057, -1058, -1060, -1059, -1061, -1060, -1059, -1061, -1057, -1060, -1062, -1060, -1060, -1060, -1057, -1060, -1057, -1060, -1059, -1060, -1060, -1061, -1060, -1059, -1060, -1059, -1057, -1062, -1058, -1062, -1056, -1059, -1059, -1061, -1058, -1061, -1058, -1059, -1061, -1059, -1061, -1059, -1059, -1059, -1061, -1058, -1059, -1057, -1058, -1060, -1062, -1060, -1058, -1060, -1061, -1060, -1059, -1057, -1059, -1060, -1059, -1058, -1059, -1064, -1061, -1061, -1059, -1061, -1059, -1060, -1061, -1058, -1060, -1057, -1060, -1060, -1058, -1059, -1059, -1059, -1060, -1059, -1060, -1062, -1061, -1059, -1059, -1059, -1059, -1060, -1061, -1058, -1060, -1059, -1057, -1059, -1060, -1060, -1062, -1061, -1060, -1058, -1063, -1058, -1060, -1062, -1061, -1058, -1060, -1060, -1059, -1061, -1060, -1061, -1059, -1060, -1056, -1059, -1060, -1060, -1059, -1060, -1060, -1060, -1060, -1059, -1060, -1059, -1060, -1060, -1060, -1059, -1061, -1062, -1060, -1059, -1059, -1062, -1058, -1057, -1062, -1059, -1060, -1059, -1058, -1058, -1057, -1061, -1060, -1061, -1058, -1061, -1059, -1059, -1060, -1060, -1060, -1057, -1058, -1060, -1062, -1057, -1057, -1059, -1061, -1060, -1060, -1059, -1060, -1060, -1058, -1060, -1061, -1060, -1060, -1059, -1062, -1060, -1060, -1062, -1060, -1060, -1059, -1062, -1059, -1061, -1059, -1062, -1059, -1059, -1059, -1060, -1062, -1061, -1061, -1060, -1061, -1062, -1058, -1064, -1061, -1059, -1060, -1060, -1063, -1061, -1060, -1057, -1062, -1062, -1061, -1060, -1062, -1060, -1062, -1057, -1061, -1061, -1058, -1061, -1061, -1059, -1061, -1057, -1060, -1060, -1060, -1060, -1060, -1060, -1061, -1060, -1060, -1060, -1060, -1061, -1059, -1059, -1060, -1056, -1061, -1060, -1057, -1059, -1061, -1060, -1062, -1059, -1056, -1056, -1061, -1060, -1057, -1059, -1060, -1058, -1059, -1060, -1059, -1060, -1060, -1060, -1061, -1060, -1060, -1057, -1058, -1059, -1057, -1061, -1058, -1062, -1060, -1057, -1061, -1061, -1060, -1061, -1059, -1062, -1057, -1061, -1058, -1061, -1058, -1057, -1060, -1060, -1059, -1060, -1060, -1057, -1062, -1059, -1060, -1061, -1058, -1059, -1060, -1061, -1059, -1060, -1058, -1059, -1060, -1059, -1060, -1059, -1061, -1060, -1058, -1060, -1061, -1060, -1058, -1059, -1060, -1060, -1060, -1060, -1061, -1061, -1062, -1058, -1061, -1061, -1060, -1059, -1059, -1059, -1059, -1060, -1061, -1059, -1059, -1059, -1059, -1061, -1060, -1060, -1060, -1058, -1061, -1060, -1056, -1060, -1058, -1060, -1061, -1060, -1061, -1063, -1058, -1057, -1059, -1060, -1062, -1062, -1061, -1061, -1060, -1060, -1061, -1060, -1061, -1060, -1063, -1058, -1059, -1058, -1060, -1058, -1055, -1061, -1061, -1059, -1058, -1060, -1061, -1061, -1059, -1062, -1060, -1060, -1061, -1060, -1061, -1060, -1061, -1059, -1060, -1059, -1058, -1060, -1059, -1062, -1061, -1058, -1061, -1060, -1062, -1059, -1059, -1060, -1061, -1062, -1058, -1061, -1060, -1060, -1060, -1059, -1060, -1063, -1059, -1060, -1061, -1060, -1062, -1061, -1061, -1062, -1059, -1057, -1062, -1065, -1059, -1061, -1058, -1061, -1061, -1059, -1060, -1058, -1060, -1061, -1060, -1059, -1060, -1059, -1063, -1062, -1059, -1064, -1060, -1061, -1061, -1062, -1058, -1060, -1061, -1060, -1059, -1059, -1061, -1057, -1059, -1060, -1058, -1060, -1060, -1062, -1060, -1059, -1061, -1061, -1059, -1060, -1060, -1059, -1060, -1057, -1060, -1057, -1060, -1060, -1060, -1059, -1059, -1061, -1060, -1060, -1059, -1060, -1058, -1060, -1060, -1063, -1063, -1061, -1060, -1059, -1061, -1058, -1060, -1061, -1059, -1059, -1060, -1063, -1063, -1058, -1061, -1060, -1057, -1061, -1060, -1059, -1061, -1058, -1062, -1058]]
  out "TraceAI6 temp":i16[](array[numeric])=[-1060, -1059, -1059, -1058, -1059, -1058, -1061, -1061, -1059, -1059, -1058, -1057, -1061, -1059, -1061, -1058, -1060, -1061, -1058, -1058, -1060, -1062, -1060, -1060, -1060, -1058, -1060, -1061, -1060, -1062, -1060, -1061, -1059, -1060, -1061, -1061, -1059, -1061, -1060, -1057, -1058, -1059, -1061, -1057, -1058, -1059, -1061, -1058, -1058, -1060, -1060, -1059, -1060, -1059, -1059, -1060, -1060, -1058, -1061, -1058, -1061, -1057, -1059, -1059, -1061, -1062, -1061, -1060, -1060, -1056, -1061, -1060, -1058, -1061, -1060, -1060, -1061, -1058, -1061, -1061, -1059, -1061, -1060, -1060, -1061, -1057, -1060, -1059, -1058, -1058, -1059, -1058, -1061, -1059, -1059, -1060, -1057, -1062, -1057, -1059, -1058, -1060, -1058, -1059, -1060, -1061, -1060, -1062, -1059, -1060, -1058, -1056, -1058, -1060, -1059, -1060, -1059, -1060, -1062, -1059, -1060, -1061, -1061, -1060, -1060, -1061, -1057, -1058, -1059, -1058, -1061, -1057, -1060, -1059, -1060, -1059, -1061, -1060, -1064, -1059, -1057, -1057, -1059, -1059, -1062, -1061, -1059, -1060, -1057, -1059, -1061, -1061, -1060, -1058, -1059, -1063, -1060, -1060, -1058, -1058, -1060, -1061, -1060, -1059, -1062, -1060, -1061, -1060, -1062, -1061, -1061, -1061, -1060, -1061, -1061, -1059, -1057, -1062, -1060, -1062, -1060, -1060, -1059, -1061, -1060, -1062, -1060, -1060, -1062, -1060, -1061, -1060, -1060, -1061, -1057, -1060, -1060, -1061, -1059, -1059, -1059, -1060, -1058, -1061, -1060, -1061, -1057, -1061, -1060, -1061, -1060, -1061, -1061, -1063, -1060, -1061, -1059, -1058, -1060, -1063, -1063, -1060, -1060, -1060, -1055, -1062, -1062, -1060, -1061, -1059, -1058, -1059, -1061, -1060, -1060, -1059, -1058, -1061, -1061, -1055, -1058, -1059, -1061, -1058, -1060, -1060, -1061, -1061, -1060, -1061, -1061, -1061, -1060, -1061, -1059, -1061, -1059, -1060, -1060, -1061, -1059, -1059, -1060, -1057, -1059, -1060, -1059, -1059, -1060, -1060, -1058, -1060, -1059, -1054, -1064, -1061, -1060, -1061, -1060, -1061, -1060, -1058, -1063, -1061, -1058, -1059, -1059, -1062, -1059, -1059, -1062, -1060, -1060, -1058, -1059, -1058, -1058, -1062, -1062, -1060, -1059, -1061, -1060, -1060, -1060, -1061, -1060, -1057, -1058, -1060, -1060, -1060, -1061, -1060, -1061, -1060, -1060, -1059, -1061, -1059, -1063, -1062, -1060, -1060, -1062, -1057, -1058, -1061, -1058, -1059, -1059, -1060, -1059, -1062, -1060, -1061, -1058, -1059, -1061, -1062, -1062, -1060, -1060, -1059, -1061, -1060, -1060, -1059, -1059, -1060, -1059, -1058, -1058, -1060, -1059, -1059, -1062, -1061, -1062, -1062, -1059, -1060, -1061, -1058, -1060, -1060, -1064, -1059, -1061, -1063, -1060, -1059, -1057, -1059, -1063, -1062, -1060, -1060, -1057, -1061, -1059, -1060, -1059, -1060, -1059, -1058, -1062, -1063, -1058, -1058, -1061, -1062, -1060, -1059, -1059, -1061, -1059, -1061, -1064, -1062, -1060, -1057, -1060, -1061, -1057, -1060, -1063, -1061, -1061, -1059, -1058, -1059, -1061, -1055, -1059, -1059, -1061, -1060, -1060, -1063, -1058, -1061, -1059, -1060, -1060, -1059, -1063, -1062, -1060, -1059, -1062, -1060, -1061, -1060, -1061, -1060, -1060, -1062, -1059, -1059, -1060, -1059, -1060, -1058, -1057, -1060, -1060, -1060, -1060, -1061, -1058, -1061, -1061, -1060, -1061, -1059, -1061, -1058, -1059, -1060, -1059, -1061, -1059, -1060, -1059, -1061, -1060, -1060, -1063, -1058, -1060, -1062, -1059, -1060, -1060, -1060, -1062, -1063, -1059, -1061, -1057, -1062, -1063, -1060, -1062, -1060, -1062, -1058, -1059, -1062, -1060, -1059, -1058, -1061, -1058, -1057, -1059, -1061, -1062, -1060, -1060, -1058, -1060, -1059, -1059, -1061, -1059, -1061, -1061, -1065, -1060, -1060]
  out "AI5 Back":i16[][](array[numeric])
  out "AI5 Array":i16[][](array[numeric])
  out "AI6 Array Back":i16[][](array[numeric])
  out "AI6 Array":i16[][](array[numeric])
  out "Internal Setpoint indicator":i16=7166
  out "iterations x":i32=83967
  out "Trace AI2 array":i16[][](array[numeric])=[[45, -178, 33, -89, -19, 26, -131, 45, -151, 10, 0, -80, 44, -182, 29, -62, -45, 30, -156, 41, -125, 2, 16, -83, 46, -175, 18, -40, -65, 39, -175, 36, -95, -12, 23, -123, 47, -156, 14, -10, -75, 47, -182, 30, -70, -36, 27, -149, 43, -136, 5, 12, -87, 48, -172, 23, -48, -58, 32, -170, 42, -107, -6, 23, -113, 48, -164, 14, -20, -71, 42, -181, 30, -79, -29, 25, -143, 45, -145, 8, 6, -84, 46, -182, 26, -57, -52, 25, -162, 34, -116, 1, 22, -104, 48, -174, 17, -30, -69, 45, -178, 33, -87, -21, 25, -133, 45, -151, 10, 0, -80, 46, -182, 27, -62, -42, 28, -156, 41, -125, 4, 16, -82, 49, -174, 23, -32, -64, 39, -175, 35, -99, -12, 23, -126, 45, -156, 14, -9, -76, 47, -181, 31, -69, -39, 26, -149, 43, -139, 8, 13, -85, 49, -169, 23, -46, -57, 30, -172, 42, -108, -6, 21, -118, 46, -165, 15, -19, -72, 43, -181, 32, -79, -29, 25, -143, 43, -145, 9, 7, -81, 47, -180, 29, -54, -53, 25, -164, 35, -116, -3, 23, -105, 49, -174, 18, -29, -69, 47, -177, 36, -86, -23, 26, -130, 44, -150, 10, 0, -77, 46, -179, 29, -60, -44, 30, -158, 38, -127, 3, 18, -82, 49, -175, 22, -32, -64, 42, -173, 37, -96, -13, 25, -127, 47, -156, 13, -8, -75, 46, -181, 33, -68, -37, 28, -150, 41, -136, 5, 12, -88, 48, -171, 24, -47, -55, 32, -171, 41, -107, -7, 24, -119, 45, -165, 16, -18, -74, 43, -182, 31, -79, -30, 28, -139, 43, -146, 8, 6, -83, 46, -179, 27, -52, -49, 27, -162, 34, -118, -1, 21, -102, 45, -174, 18, -31, -69, 47, -176, 36, -86, -20, 27, -132, 46, -152, 9, -1, -79, 48, -180, 27, -62, -42, 29, -155, 39, -126, 4, 16, -83, 48, -174, 22, -35, -65, 43, -173, 37, -96, -12, 23, -124, 46, -160, 12, -7, -74, 44, -181, 32, -67, -37, 29, -146, 42, -136, 4, 12, -87, 47, -172, 24, -46, -56, 31, -168, 42, -106, -6, 22, -113, 48, -164, 14, -20, -71, 43, -178, 31, -78, -28, 28, -140, 44, -143, 9, 7, -83, 48, -181, 27, -56, -50, 27, -163, 35, -116, 0, 20, -104, 47, -174, 19, -30, -67, 46, -176, 33, -87, -18, 27, -130, 46, -150, 11, 0, -78, 46, -182, 27, -63, -42, 30, -158, 42, -127, 3, 16, -81, 49, -174, 19, -41, -65, 40, -173, 35, -99, -12, 25, -126, 45, -159, 12, -9, -76, 46, -183, 33, -72, -36, 27, -149, 42, -137, 5, 13, -86, 48, -171, 23, -51, -57, 28, -169, 41, -108, -5, 24, -114, 48, -165, 17, -21, -73, 42, -180, 31, -78, -30, 26, -142, 43, -145, 9, 5, -81, 49, -178, 25, -57, -51, 27, -164, 36, -120, 0, 19, -100, 49, -175, 18, -32, -71, 45, -178, 32, -89, -19, 26, -129, 47, -149, 12, -2, -79, 47, -180, 27, -62, -44], [-82, 32, -177, 42, -72, -22, 15, -169, 47, -110, 22, -6, -112, 42, -169, 27, -55, -49, -62, 28, -182, 45, -77, 0, 10, -153, 46, -133, 26, -22, -87, 36, -177, 47, -66, -30, 17, -173, 46, -103, 19, -1, -118, 34, -165, 26, -51, -53, 25, -179, 46, -81, 6, 9, -146, 43, -140, 24, -29, -80, 32, -181, 43, -71, -21, 17, -165, 46, -115, 24, -5, -108, 39, -168, 30, -56, -48, 23, -174, 47, -87, 12, 6, -138, 42, -149, 28, -37, -70, 32, -180, 45, -73, -9, 15, -160, 46, -126, 24, -13, -98, 40, -174, 40, -65, -39, 21, -170, 48, -82, 16, 3, -128, 40, -158, 30, -43, -62, 29, -179, 46, -77, 1, 12, -151, 44, -129, 24, -18, -90, 34, -177, 47, -67, -30, 18, -174, 46, -100, 21, 1, -118, 34, -162, 24, -51, -56, 27, -179, 49, -81, 6, 8, -146, 42, -141, 26, -28, -80, 33, -181, 40, -73, -20, 16, -165, 48, -117, 23, -8, -110, 42, -172, 27, -57, -49, 22, -173, 48, -86, 13, 7, -137, 43, -146, 27, -39, -71, 29, -182, 46, -75, -10, 12, -157, 45, -126, 24, -11, -100, 34, -174, 39, -63, -44, 20, -170, 50, -80, 17, 6, -131, 42, -159, 27, -43, -65, 27, -181, 45, -79, -2, 9, -153, 46, -128, 23, -18, -88, 34, -177, 45, -68, -31, 17, -176, 50, -99, 22, 1, -118, 35, -161, 29, -50, -54, 27, -182, 47, -84, 6, 9, -146, 44, -140, 26, -29, -80, 33, -179, 42, -71, -23, 18, -163, 47, -111, 23, -3, -110, 42, -168, 29, -55, -49, 22, -175, 46, -87, 12, 6, -137, 44, -149, 27, -35, -69, 31, -183, 44, -75, -11, 13, -161, 46, -123, 25, -12, -98, 38, -172, 39, -63, -40, 21, -174, 48, -84, 17, 5, -130, 40, -154, 29, -44, -64, 28, -182, 45, -79, 0, 10, -153, 46, -129, 27, -17, -87, 34, -175, 46, -68, -31, 19, -175, 47, -101, 21, 1, -117, 36, -161, 28, -48, -55, 26, -181, 47, -83, 5, 8, -148, 45, -140, 26, -26, -78, 32, -176, 43, -71, -22, 17, -168, 47, -110, 24, -5, -109, 41, -169, 26, -54, -49, 25, -173, 48, -85, 10, 4, -137, 42, -146, 27, -32, -69, 32, -180, 45, -74, -10, 13, -160, 45, -128, 22, -12, -100, 38, -172, 42, -62, -41, 21, -170, 48, -81, 16, 5, -131, 41, -155, 29, -41, -64, 29, -181, 48, -77, -1, 10, -152, 45, -132, 24, -19, -90, 36, -175, 45, -67, -30, 20, -176, 48, -99, 18, 1, -119, 36, -161, 27, -51, -56, 27, -180, 48, -81, 6, 9, -147, 43, -139, 24, -28, -81, 33, -179, 43, -71, -23, 16, -166, 46, -108, 22, -4, -111, 41, -168, 27, -57, -50, 25, -174, 49, -86, 9, 4, -137, 44, -147, 26, -36, -72, 32, -181, 47, -75, -10, 14, -160, 46, -125, 23, -10, -99, 39, -174, 39, -64, -41, 22, -171, 49, -81, 16, 3, -128, 43, -158, 31]]
  out "TraceAI2 array temp":i16[](array[numeric])=[-26, 25, -140, 43, -150, 7, 3, -83, 46, -180, 28, -55, -49, 28, -163, 35, -121, 1, 19, -98, 48, -178, 19, -33, -69, 46, -178, 35, -90, -17, 24, -128, 44, -157, 9, -4, -79, 46, -182, 30, -63, -41, 30, -155, 41, -130, 3, 14, -83, 49, -169, 23, -45, -63, 40, -173, 39, -99, -10, 24, -126, 44, -164, 13, -13, -77, 44, -181, 32, -72, -33, 28, -144, 43, -137, 5, 9, -88, 47, -178, 22, -52, -55, 27, -168, 42, -111, -5, 23, -109, 48, -166, 15, -23, -71, 43, -182, 31, -82, -30, 25, -139, 44, -149, 10, 4, -81, 47, -182, 28, -58, -51, 29, -161, 36, -118, 2, 19, -95, 47, -178, 17, -34, -69, 47, -177, 33, -90, -19, 25, -131, 47, -154, 11, -2, -79, 45, -184, 28, -63, -42, 29, -155, 43, -131, 6, 17, -80, 47, -170, 19, -43, -65, 39, -175, 38, -99, -10, 23, -123, 47, -162, 14, -10, -75, 46, -182, 31, -72, -35, 27, -149, 43, -140, 5, 11, -85, 46, -174, 21, -50, -58, 27, -170, 41, -110, -4, 23, -113, 49, -165, 16, -20, -72, 43, -182, 31, -78, -30, 25, -140, 44, -147, 9, 4, -80, 47, -181, 26, -55, -50, 28, -161, 35, -118, 1, 20, -100, 49, -175, 18, -30, -69, 44, -178, 34, -88, -21, 26, -132, 45, -152, 11, -2, -77, 48, -182, 30, -62, -43, 29, -157, 41, -128, 4, 17, -81, 50, -172, 22, -38, -62, 40, -174, 37, -98, -13, 23, -122, 46, -158, 13, -10, -75, 47, -182, 33, -71, -37, 27, -148, 41, -136, 7, 13, -84, 48, -172, 24, -46, -56, 31, -170, 40, -107, -7, 24, -116, 47, -165, 16, -18, -72, 43, -181, 34, -79, -30, 26, -141, 43, -145, 9, 7, -82, 47, -178, 26, -55, -51, 27, -165, 35, -117, 1, 21, -101, 47, -174, 19, -29, -67, 46, -178, 35, -85, -22, 24, -134, 44, -151, 11, 0, -80, 46, -180, 28, -62, -45, 29, -159, 40, -126, 3, 16, -83, 48, -175, 22, -37, -64, 40, -175, 35, -97, -13, 25, -127, 46, -158, 13, -8, -77, 47, -179, 33, -67, -37, 26, -152, 44, -137, 5, 13, -86, 48, -172, 23, -46, -57, 36, -171, 40, -108, -7, 22, -122, 45, -168, 15, -18, -73, 45, -183, 31, -74, -32, 26, -143, 43, -146, 8, 8, -85, 48, -179, 26, -51, -51, 24, -164, 36, -115, -3, 20, -107, 47, -173, 19, -27, -69, 46, -177, 35, -86, -23, 26, -135, 41, -152, 8, 0, -80, 45, -180, 27, -60, -44, 31, -158, 38, -123, 1, 18, -86, 48, -177, 19, -36, -66, 42, -176, 35, -92, -16, 24, -126, 48, -158, 11, -5, -78, 48, -181, 30, -67, -40, 30, -151, 42, -132, 4, 13, -86, 46, -169, 22, -46, -60, 39, -170, 41, -102, -9, 23, -126, 47, -165, 13, -15, -73, 42, -181, 31, -73, -34, 30, -144, 43, -141, 7, 8, -87, 47, -181, 24, -51, -56, 27, -167, 41, -111]
  out "Trace Topography Array":i32[][](array[numeric])=[[2578410, 2578426, 2578418, 2578413, 2578392, 2578366, 2578366, 2578368, 2578377, 2578391, 2578393, 2578372, 2578349, 2578326, 2578333, 2578351, 2578378, 2578397, 2578411, 2578417, 2578388, 2578381, 2578388, 2578373, 2578375, 2578370, 2578352, 2578351, 2578349, 2578349, 2578329, 2578325, 2578341, 2578362, 2578357, 2578378, 2578397, 2578402, 2578414, 2578425, 2578437, 2578433, 2578422, 2578434, 2578407, 2578414, 2578430, 2578435, 2578443, 2578426, 2578435, 2578433, 2578438, 2578465, 2578492, 2578523, 2578533, 2578536, 2578545, 2578550, 2578565, 2578583, 2578580, 2578579, 2578566, 2578544, 2578562, 2578565, 2578572, 2578582, 2578597, 2578618, 2578638, 2578657, 2578673, 2578683, 2578690, 2578698, 2578703, 2578712, 2578717, 2578698, 2578699, 2578665, 2578667, 2578658, 2578648, 2578649, 2578647, 2578657, 2578677, 2578696, 2578724, 2578728, 2578751, 2578768, 2578763, 2578775, 2578766, 2578759, 2578740, 2578730, 2578721, 2578706, 2578697, 2578700, 2578690, 2578698, 2578720, 2578756, 2578789, 2578820, 2578841, 2578862, 2578864, 2578874, 2578873, 2578860, 2578848, 2578842, 2578831, 2578816, 2578809, 2578805, 2578792, 2578810, 2578816, 2578829, 2578835, 2578849, 2578857, 2578876, 2578897, 2578902, 2578900, 2578883, 2578874, 2578870, 2578834, 2578846, 2578835, 2578828, 2578827, 2578831, 2578846, 2578850, 2578877, 2578915, 2578931, 2578946, 2578962, 2578968, 2578971, 2578983, 2578991, 2578992, 2578978, 2578977, 2578989, 2578989, 2578998, 2579005, 2579001, 2579015, 2579038, 2579045, 2579071, 2579105, 2579131, 2579147, 2579175, 2579192, 2579208, 2579225, 2579238, 2579251, 2579258, 2579279, 2579290, 2579297, 2579301, 2579302, 2579308, 2579314, 2579324, 2579326, 2579329, 2579347, 2579375, 2579402, 2579418, 2579429, 2579443, 2579444, 2579450, 2579455, 2579465, 2579471, 2579491, 2579482, 2579492, 2579488, 2579502, 2579499, 2579515, 2579530, 2579544, 2579549, 2579534, 2579526, 2579526, 2579522, 2579545, 2579568, 2579564, 2579575, 2579577, 2579579, 2579597, 2579618, 2579650, 2579664, 2579654, 2579657, 2579668, 2579654, 2579678, 2579682, 2579677, 2579694, 2579690, 2579699, 2579706, 2579718, 2579727, 2579724, 2579747, 2579761, 2579796, 2579808, 2579832, 2579856, 2579848, 2579848, 2579835, 2579829, 2579835, 2579830, 2579830, 2579846, 2579864, 2579861, 2579869, 2579887, 2579908, 2579921, 2579930, 2579953, 2579969, 2579992, 2580010, 2580008, 2580022, 2580019, 2580020, 2580003, 2580015, 2580029, 2580023, 2580034, 2580054, 2580053, 2580054, 2580058, 2580074, 2580090, 2580115, 2580122, 2580131, 2580130, 2580151, 2580158, 2580161, 2580166, 2580163, 2580161, 2580170, 2580186, 2580198, 2580217, 2580219, 2580227, 2580251, 2580281, 2580286, 2580303, 2580310, 2580295, 2580289, 2580299, 2580294, 2580300, 2580305, 2580304, 2580312, 2580310, 2580309, 2580323, 2580346, 2580363, 2580395, 2580394, 2580403, 2580398, 2580419, 2580429, 2580447, 2580469, 2580471, 2580479, 2580494, 2580491, 2580506, 2580516, 2580508, 2580510, 2580513, 2580500, 2580520, 2580526, 2580555, 2580560, 2580568, 2580600, 2580602, 2580614, 2580613, 2580607, 2580609, 2580605, 2580607, 2580621, 2580608, 2580614, 2580618, 2580613, 2580637, 2580672, 2580683, 2580696, 2580710, 2580742, 2580750, 2580767, 2580789, 2580792, 2580809, 2580836, 2580822, 2580820, 2580823, 2580825, 2580825, 2580826, 2580821, 2580815, 2580837, 2580847, 2580852, 2580839, 2580852, 2580861, 2580879, 2580895, 2580915, 2580946, 2580960, 2580982, 2580991, 2580993, 2581001, 2581003, 2581005, 2581008, 2581024, 2581036, 2581036, 2581038, 2581029, 2581013, 2581017, 2581035, 2581057, 2581081, 2581103, 2581111, 2581118, 2581123, 2581130, 2581162, 2581186, 2581204, 2581198, 2581201, 2581200, 2581203, 2581243, 2581267, 2581284, 2581288, 2581268, 2581256, 2581248, 2581248, 2581252, 2581271, 2581281, 2581295, 2581280, 2581297, 2581312, 2581331, 2581346, 2581358, 2581373, 2581394, 2581410, 2581410, 2581413, 2581440, 2581456, 2581439, 2581449, 2581465, 2581464, 2581474, 2581469, 2581476, 2581489, 2581502, 2581513, 2581517, 2581532, 2581534, 2581538, 2581538, 2581547, 2581553, 2581554, 2581566, 2581577, 2581577, 2581582, 2581601, 2581617, 2581635, 2581639, 2581631, 2581632, 2581636, 2581643, 2581670, 2581686, 2581687, 2581695, 2581695, 2581706, 2581714, 2581736, 2581749, 2581748, 2581750, 2581767, 2581774, 2581769, 2581774, 2581775, 2581781, 2581767, 2581781, 2581797, 2581827, 2581838, 2581837, 2581859, 2581862, 2581861, 2581858, 2581883, 2581900, 2581918, 2581917, 2581928, 2581964, 2581976, 2582013, 2582004, 2582004, 2581998, 2581967, 2581970, 2581978, 2581980, 2581986, 2581999, 2581994, 2581987, 2581992, 2582001, 2582011, 2582026, 2582035], [2578296, 2578308, 2578305, 2578316, 2578335, 2578347, 2578370, 2578369, 2578388, 2578405, 2578431, 2578437, 2578452, 2578453, 2578460, 2578460, 2578464, 2578457, 2578470, 2578490, 2578495, 2578510, 2578506, 2578505, 2578515, 2578519, 2578522, 2578518, 2578542, 2578565, 2578576, 2578601, 2578619, 2578616, 2578619, 2578637, 2578652, 2578656, 2578632, 2578634, 2578629, 2578619, 2578631, 2578637, 2578641, 2578630, 2578619, 2578625, 2578635, 2578669, 2578688, 2578694, 2578705, 2578707, 2578722, 2578736, 2578744, 2578751, 2578737, 2578742, 2578746, 2578747, 2578752, 2578772, 2578785, 2578786, 2578780, 2578783, 2578788, 2578782, 2578795, 2578813, 2578815, 2578839, 2578839, 2578835, 2578838, 2578859, 2578874, 2578893, 2578912, 2578921, 2578930, 2578939, 2578936, 2578943, 2578966, 2579002, 2579023, 2579033, 2579051, 2579059, 2579052, 2579050, 2579069, 2579070, 2579077, 2579087, 2579091, 2579101, 2579093, 2579113, 2579120, 2579126, 2579137, 2579149, 2579157, 2579164, 2579175, 2579185, 2579182, 2579162, 2579155, 2579132, 2579145, 2579158, 2579148, 2579154, 2579154, 2579162, 2579155, 2579148, 2579156, 2579175, 2579178, 2579202, 2579216, 2579217, 2579223, 2579234, 2579241, 2579258, 2579266, 2579275, 2579255, 2579263, 2579267, 2579277, 2579289, 2579312, 2579319, 2579329, 2579321, 2579332, 2579330, 2579330, 2579337, 2579345, 2579367, 2579372, 2579355, 2579367, 2579379, 2579386, 2579388, 2579382, 2579391, 2579400, 2579391, 2579388, 2579382, 2579386, 2579387, 2579403, 2579419, 2579422, 2579433, 2579422, 2579435, 2579469, 2579492, 2579511, 2579549, 2579578, 2579577, 2579597, 2579618, 2579641, 2579655, 2579675, 2579700, 2579717, 2579740, 2579760, 2579778, 2579796, 2579813, 2579813, 2579814, 2579833, 2579856, 2579878, 2579891, 2579891, 2579891, 2579881, 2579882, 2579890, 2579889, 2579896, 2579901, 2579922, 2579935, 2579933, 2579957, 2579965, 2579977, 2579989, 2579993, 2580012, 2580009, 2580017, 2580022, 2580034, 2580035, 2580036, 2580032, 2580042, 2580060, 2580072, 2580084, 2580090, 2580110, 2580117, 2580136, 2580128, 2580132, 2580151, 2580155, 2580169, 2580149, 2580149, 2580146, 2580148, 2580151, 2580151, 2580153, 2580159, 2580185, 2580190, 2580184, 2580191, 2580205, 2580221, 2580250, 2580262, 2580271, 2580278, 2580298, 2580298, 2580308, 2580317, 2580322, 2580349, 2580352, 2580373, 2580384, 2580392, 2580393, 2580392, 2580407, 2580423, 2580418, 2580413, 2580418, 2580411, 2580419, 2580413, 2580412, 2580419, 2580422, 2580439, 2580436, 2580447, 2580467, 2580480, 2580489, 2580503, 2580517, 2580534, 2580545, 2580561, 2580570, 2580563, 2580570, 2580580, 2580577, 2580591, 2580588, 2580583, 2580602, 2580608, 2580606, 2580620, 2580612, 2580618, 2580624, 2580644, 2580674, 2580675, 2580699, 2580705, 2580707, 2580715, 2580726, 2580722, 2580719, 2580716, 2580725, 2580725, 2580753, 2580771, 2580776, 2580773, 2580780, 2580794, 2580792, 2580802, 2580816, 2580816, 2580816, 2580842, 2580858, 2580865, 2580879, 2580883, 2580899, 2580907, 2580900, 2580905, 2580919, 2580922, 2580936, 2580939, 2580962, 2580980, 2581011, 2581018, 2581015, 2581021, 2581036, 2581049, 2581058, 2581069, 2581072, 2581069, 2581064, 2581075, 2581068, 2581068, 2581089, 2581086, 2581105, 2581112, 2581118, 2581137, 2581155, 2581174, 2581197, 2581209, 2581211, 2581230, 2581248, 2581254, 2581273, 2581267, 2581254, 2581242, 2581240, 2581248, 2581253, 2581274, 2581272, 2581265, 2581276, 2581272, 2581284, 2581291, 2581304, 2581331, 2581341, 2581347, 2581342, 2581335, 2581336, 2581347, 2581351, 2581356, 2581363, 2581380, 2581384, 2581404, 2581429, 2581439, 2581469, 2581482, 2581483, 2581486, 2581478, 2581477, 2581456, 2581443, 2581434, 2581422, 2581429, 2581426, 2581434, 2581446, 2581449, 2581449, 2581492, 2581511, 2581525, 2581550, 2581566, 2581570, 2581578, 2581591, 2581604, 2581600, 2581595, 2581606, 2581615, 2581618, 2581613, 2581608, 2581626, 2581622, 2581629, 2581654, 2581686, 2581714, 2581736, 2581761, 2581764, 2581759, 2581760, 2581760, 2581755, 2581769, 2581771, 2581756, 2581755, 2581751, 2581759, 2581755, 2581750, 2581757, 2581753, 2581758, 2581779, 2581804, 2581820, 2581846, 2581850, 2581846, 2581845, 2581849, 2581836, 2581834, 2581830, 2581814, 2581845, 2581859, 2581872, 2581895, 2581894, 2581902, 2581916, 2581939, 2581949, 2581966, 2581976, 2581997, 2582004, 2582021, 2582021, 2582019, 2582019, 2582011, 2581998, 2582005, 2581989, 2581990, 2581994, 2581994, 2582011, 2581993, 2581993, 2581988, 2581985, 2581987, 2581990, 2582004, 2581993, 2582006, 2582016, 2582049, 2582067, 2582092, 2582101, 2582097, 2582091, 2582083, 2582079, 2582069, 2582071, 2582056, 2582049, 2582044, 2582033, 2582029]]
  out "Trace Topography Array temp":i32[](array[numeric])=[2578273, 2578265, 2578249, 2578244, 2578242, 2578236, 2578264, 2578277, 2578285, 2578291, 2578290, 2578284, 2578284, 2578284, 2578294, 2578294, 2578315, 2578302, 2578286, 2578284, 2578290, 2578299, 2578317, 2578333, 2578349, 2578362, 2578357, 2578366, 2578359, 2578377, 2578374, 2578365, 2578381, 2578376, 2578381, 2578390, 2578390, 2578384, 2578386, 2578383, 2578392, 2578401, 2578402, 2578406, 2578420, 2578418, 2578411, 2578418, 2578418, 2578412, 2578417, 2578429, 2578457, 2578473, 2578488, 2578484, 2578488, 2578493, 2578481, 2578481, 2578475, 2578476, 2578488, 2578491, 2578514, 2578519, 2578543, 2578556, 2578540, 2578532, 2578518, 2578513, 2578520, 2578501, 2578513, 2578517, 2578538, 2578559, 2578574, 2578593, 2578603, 2578610, 2578627, 2578622, 2578637, 2578642, 2578631, 2578634, 2578621, 2578619, 2578603, 2578592, 2578583, 2578593, 2578587, 2578588, 2578582, 2578582, 2578599, 2578609, 2578636, 2578660, 2578689, 2578704, 2578709, 2578721, 2578723, 2578724, 2578713, 2578705, 2578701, 2578705, 2578683, 2578692, 2578704, 2578722, 2578737, 2578751, 2578765, 2578765, 2578764, 2578784, 2578778, 2578775, 2578777, 2578762, 2578745, 2578746, 2578742, 2578737, 2578736, 2578740, 2578751, 2578757, 2578771, 2578787, 2578800, 2578829, 2578828, 2578848, 2578835, 2578828, 2578833, 2578829, 2578816, 2578829, 2578826, 2578838, 2578842, 2578838, 2578848, 2578846, 2578843, 2578859, 2578881, 2578902, 2578929, 2578933, 2578965, 2578987, 2578999, 2579008, 2579023, 2579021, 2579010, 2579022, 2579029, 2579014, 2579019, 2579027, 2579028, 2579056, 2579065, 2579079, 2579100, 2579122, 2579137, 2579155, 2579174, 2579214, 2579205, 2579222, 2579222, 2579204, 2579201, 2579199, 2579207, 2579211, 2579230, 2579241, 2579237, 2579240, 2579254, 2579280, 2579301, 2579328, 2579344, 2579368, 2579387, 2579388, 2579396, 2579390, 2579390, 2579382, 2579353, 2579367, 2579362, 2579372, 2579376, 2579364, 2579372, 2579390, 2579394, 2579428, 2579435, 2579458, 2579471, 2579470, 2579499, 2579496, 2579505, 2579523, 2579503, 2579500, 2579490, 2579498, 2579513, 2579511, 2579519, 2579534, 2579547, 2579576, 2579601, 2579615, 2579637, 2579639, 2579646, 2579666, 2579677, 2579693, 2579679, 2579691, 2579687, 2579678, 2579680, 2579674, 2579692, 2579698, 2579710, 2579709, 2579707, 2579712, 2579725, 2579725, 2579745, 2579753, 2579765, 2579801, 2579807, 2579803, 2579799, 2579805, 2579819, 2579826, 2579830, 2579845, 2579848, 2579834, 2579847, 2579833, 2579829, 2579827, 2579824, 2579845, 2579863, 2579879, 2579887, 2579886, 2579918, 2579932, 2579947, 2579958, 2579973, 2579958, 2579969, 2579967, 2579970, 2579988, 2579983, 2579994, 2579986, 2579993, 2580022, 2580036, 2580038, 2580063, 2580076, 2580084, 2580091, 2580103, 2580128, 2580136, 2580150, 2580143, 2580144, 2580147, 2580148, 2580166, 2580150, 2580151, 2580160, 2580166, 2580164, 2580186, 2580197, 2580210, 2580219, 2580234, 2580240, 2580244, 2580268, 2580282, 2580302, 2580304, 2580295, 2580281, 2580286, 2580307, 2580322, 2580341, 2580354, 2580347, 2580351, 2580360, 2580366, 2580383, 2580395, 2580393, 2580400, 2580398, 2580400, 2580405, 2580399, 2580413, 2580402, 2580408, 2580409, 2580400, 2580401, 2580420, 2580431, 2580442, 2580460, 2580467, 2580483, 2580492, 2580498, 2580503, 2580497, 2580512, 2580504, 2580497, 2580506, 2580511, 2580504, 2580503, 2580510, 2580524, 2580531, 2580535, 2580545, 2580546, 2580565, 2580580, 2580586, 2580607, 2580613, 2580611, 2580621, 2580647, 2580663, 2580669, 2580674, 2580689, 2580662, 2580655, 2580657, 2580654, 2580654, 2580664, 2580675, 2580674, 2580665, 2580694, 2580713, 2580730, 2580762, 2580774, 2580801, 2580830, 2580835, 2580842, 2580837, 2580842, 2580842, 2580837, 2580844, 2580843, 2580834, 2580843, 2580834, 2580858, 2580862, 2580880, 2580901, 2580904, 2580916, 2580925, 2580944, 2580964, 2580969, 2580978, 2581002, 2580996, 2580990, 2580988, 2581003, 2581020, 2581028, 2581037, 2581060, 2581061, 2581064, 2581082, 2581071, 2581082, 2581079, 2581076, 2581068, 2581068, 2581066, 2581071, 2581080, 2581096, 2581102, 2581111, 2581141, 2581148, 2581170, 2581197, 2581233, 2581240, 2581238, 2581236, 2581234, 2581217, 2581237, 2581256, 2581254, 2581265, 2581265, 2581265, 2581259, 2581258, 2581284, 2581281, 2581298, 2581308, 2581344, 2581358, 2581368, 2581383, 2581398, 2581403, 2581417, 2581405, 2581396, 2581397, 2581373, 2581376, 2581373, 2581371, 2581370, 2581372, 2581365, 2581375, 2581377, 2581387, 2581409, 2581421, 2581456, 2581474, 2581468, 2581481, 2581487, 2581503, 2581506, 2581500, 2581509, 2581515, 2581509, 2581491, 2581493, 2581491, 2581507, 2581511, 2581509, 2581513, 2581523, 2581533, 2581530, 2581535]
  out "Trace AI0 Array":i16[][](array[numeric])=[[80, -305, 87, -353, 20, 35, -176, 95, -394, 58, -111, -77, 89, -347, 82, -308, -11, 55, -233, 92, -393, 51, -27, -96, 94, -378, 71, -240, -45, 74, -282, 87, -365, 33, 25, -159, 95, -391, 61, -146, -67, 87, -335, 80, -324, -3, 51, -215, 94, -395, 51, -49, -95, 93, -363, 76, -273, -34, 62, -277, 93, -374, 38, 13, -137, 95, -389, 65, -183, -59, 82, -320, 82, -340, 9, 40, -192, 95, -401, 55, -82, -87, 91, -362, 77, -292, -24, 57, -250, 87, -385, 45, -5, -123, 96, -392, 66, -221, -53, 80, -304, 86, -356, 21, 30, -178, 94, -395, 57, -113, -78, 87, -346, 78, -308, -12, 55, -234, 89, -392, 50, -26, -96, 94, -379, 72, -236, -43, 71, -286, 87, -369, 31, 22, -160, 94, -395, 62, -149, -69, 85, -341, 82, -328, -2, 46, -213, 92, -395, 52, -56, -98, 92, -363, 76, -269, -32, 64, -272, 91, -377, 38, 15, -145, 93, -390, 63, -181, -61, 82, -321, 82, -341, 10, 41, -197, 92, -398, 56, -80, -84, 91, -358, 77, -288, -24, 53, -254, 87, -385, 45, -4, -126, 95, -390, 67, -217, -54, 82, -304, 86, -353, 20, 33, -175, 95, -397, 58, -110, -74, 89, -350, 79, -311, -13, 54, -234, 92, -391, 48, -27, -92, 91, -378, 72, -243, -43, 72, -291, 87, -366, 30, 23, -163, 96, -390, 60, -146, -68, 87, -336, 82, -324, 0, 51, -216, 92, -396, 53, -51, -95, 94, -361, 75, -272, -33, 62, -268, 90, -378, 36, 13, -143, 94, -389, 64, -181, -63, 81, -323, 86, -343, 9, 41, -197, 93, -390, 57, -80, -87, 91, -358, 79, -295, -23, 55, -252, 86, -386, 43, -9, -120, 97, -390, 67, -221, -51, 79, -304, 87, -355, 22, 33, -178, 93, -400, 59, -111, -79, 90, -348, 78, -310, -11, 55, -232, 92, -391, 46, -26, -92, 95, -375, 69, -233, -45, 73, -285, 90, -366, 32, 26, -159, 95, -395, 62, -148, -71, 85, -338, 84, -325, -2, 49, -215, 93, -398, 54, -52, -93, 93, -360, 72, -276, -33, 62, -271, 91, -378, 42, 14, -142, 96, -389, 67, -185, -62, 81, -323, 83, -339, 9, 39, -195, 93, -396, 55, -79, -87, 90, -365, 78, -294, -25, 56, -251, 86, -384, 45, -7, -117, 93, -388, 68, -216, -52, 81, -303, 84, -354, 22, 33, -172, 93, -394, 60, -118, -77, 89, -344, 80, -308, -11, 53, -231, 90, -391, 50, -29, -88, 95, -375, 70, -254, -47, 74, -281, 91, -371, 31, 25, -156, 97, -393, 63, -149, -69, 86, -331, 81, -327, 0, 49, -214, 92, -396, 55, -54, -94, 91, -361, 75, -272, -31, 59, -272, 91, -377, 42, 12, -140, 96, -388, 66, -189, -61, 83, -314, 83, -342, 11, 40, -194, 92, -397, 55, -84, -81, 92, -358, 77, -293, -20, 55, -252, 87, -387, 47, -6, -116, 96, -389, 68, -225, -52, 78, -302, 86, -356, 23, 34, -169, 95, -396, 60, -120, -76, 87, -347, 80, -310, -7], [-342, 80, -313, 82, -58, -196, 66, -389, 96, -132, 5, 45, -377, 90, -264, 59, -27, -280, -311, 76, -349, 88, -76, -113, 57, -396, 94, -175, 34, 18, -351, 85, -305, 82, -53, -219, 69, -386, 94, -123, -5, 44, -386, 86, -254, 53, -21, -292, 76, -361, 89, -83, -83, 55, -399, 95, -192, 39, 11, -342, 83, -319, 80, -54, -185, 68, -389, 93, -136, 11, 40, -377, 89, -270, 62, -31, -274, 76, -359, 92, -94, -52, 54, -396, 92, -213, 46, 3, -328, 81, -333, 85, -69, -151, 64, -393, 94, -159, 19, 31, -371, 89, -288, 71, -43, -249, 70, -370, 95, -88, -28, 51, -391, 91, -231, 55, -7, -307, 80, -347, 88, -74, -114, 60, -391, 97, -175, 35, 22, -355, 87, -302, 81, -53, -226, 68, -387, 94, -110, -6, 46, -385, 86, -249, 54, -20, -294, 77, -356, 90, -85, -84, 56, -394, 95, -191, 39, 11, -340, 83, -316, 80, -60, -187, 64, -388, 96, -138, 10, 39, -378, 91, -270, 61, -34, -270, 72, -357, 92, -92, -56, 52, -396, 92, -212, 50, 2, -327, 84, -331, 87, -69, -155, 61, -393, 95, -154, 25, 36, -367, 89, -291, 72, -42, -252, 71, -371, 93, -93, -29, 51, -393, 94, -231, 53, -10, -313, 80, -344, 88, -75, -111, 60, -394, 95, -166, 32, 23, -355, 86, -301, 79, -50, -222, 69, -388, 95, -116, -7, 46, -384, 87, -248, 56, -21, -294, 77, -357, 93, -82, -88, 58, -391, 93, -193, 40, 11, -343, 83, -316, 84, -59, -191, 67, -386, 96, -137, 11, 40, -379, 92, -269, 59, -31, -275, 73, -359, 93, -93, -53, 52, -397, 92, -212, 48, -1, -326, 82, -331, 86, -65, -152, 60, -390, 94, -158, 23, 36, -366, 90, -282, 72, -42, -250, 73, -369, 93, -92, -28, 49, -393, 91, -228, 55, -9, -312, 79, -341, 88, -75, -115, 58, -394, 93, -174, 32, 22, -352, 86, -302, 78, -49, -219, 67, -387, 93, -115, -5, 45, -386, 89, -245, 54, -16, -288, 79, -355, 91, -85, -83, 55, -397, 97, -191, 40, 12, -341, 83, -321, 81, -59, -191, 64, -387, 94, -131, 10, 40, -377, 92, -266, 59, -29, -274, 75, -360, 91, -87, -63, 51, -395, 93, -211, 47, 1, -326, 84, -331, 85, -67, -155, 62, -390, 96, -157, 21, 32, -369, 88, -285, 72, -40, -254, 70, -368, 95, -91, -29, 51, -399, 92, -231, 50, -10, -312, 79, -346, 87, -73, -119, 58, -396, 95, -172, 32, 24, -361, 86, -297, 79, -50, -227, 67, -388, 94, -117, -11, 49, -385, 87, -249, 53, -16, -295, 77, -355, 89, -78, -83, 56, -397, 94, -193, 41, 12, -344, 86, -315, 82, -63, -189, 65, -388, 95, -131, 11, 39, -379, 88, -269, 57, -28, -275, 76, -361, 90, -90, -55, 55, -393, 93, -210, 48, 3, -327, 82, -330, 86, -67, -154, 62, -392, 94, -156, 23, 35, -363, 88, -282, 72, -42, -251, 70, -372, 95, -89, -30, 50, -393, 92, -232, 55]]
  out "Trace AI0 array temp":i16[](array[numeric])=[12, 37, -191, 94, -398, 58, -90, -81, 91, -356, 77, -298, -18, 58, -246, 88, -389, 49, -11, -113, 95, -389, 69, -231, -50, 80, -299, 84, -360, 26, 30, -169, 94, -395, 59, -123, -74, 87, -342, 80, -315, -7, 49, -228, 93, -395, 49, -33, -95, 95, -368, 69, -257, -42, 70, -282, 87, -370, 36, 20, -152, 93, -391, 64, -160, -65, 85, -330, 83, -330, 5, 45, -206, 93, -395, 53, -59, -94, 92, -362, 75, -280, -27, 58, -267, 91, -375, 45, 9, -132, 96, -388, 65, -193, -59, 81, -318, 83, -347, 12, 38, -189, 94, -398, 56, -89, -81, 89, -354, 78, -295, -20, 54, -247, 87, -388, 46, -11, -112, 94, -387, 68, -224, -48, 79, -302, 85, -353, 27, 30, -170, 94, -395, 58, -117, -75, 88, -345, 77, -314, -8, 52, -231, 90, -394, 49, -32, -94, 93, -370, 73, -254, -44, 70, -285, 90, -367, 31, 19, -156, 95, -393, 62, -155, -65, 84, -329, 83, -324, -3, 45, -211, 93, -395, 53, -56, -92, 91, -364, 74, -276, -31, 59, -272, 90, -379, 41, 9, -134, 96, -391, 65, -192, -60, 82, -319, 82, -343, 16, 40, -192, 94, -398, 55, -85, -82, 92, -359, 77, -296, -20, 55, -250, 86, -385, 45, -8, -117, 95, -390, 68, -220, -53, 81, -301, 86, -354, 21, 32, -173, 95, -397, 58, -108, -80, 87, -344, 81, -316, -6, 55, -231, 94, -391, 52, -29, -92, 96, -374, 69, -249, -42, 72, -289, 88, -367, 32, 21, -156, 96, -393, 61, -149, -67, 86, -334, 80, -326, 1, 48, -212, 92, -398, 54, -49, -91, 93, -360, 75, -276, -30, 59, -274, 89, -379, 41, 11, -139, 95, -390, 67, -186, -61, 83, -323, 87, -340, 8, 40, -195, 95, -397, 56, -79, -87, 89, -357, 77, -287, -22, 57, -251, 88, -388, 49, -5, -120, 93, -389, 69, -220, -52, 80, -303, 84, -356, 21, 29, -178, 96, -399, 56, -113, -74, 89, -350, 79, -310, -10, 48, -235, 91, -391, 49, -26, -98, 94, -377, 72, -246, -45, 75, -289, 89, -367, 30, 27, -160, 94, -392, 60, -143, -69, 86, -337, 82, -320, 0, 51, -216, 92, -394, 53, -48, -95, 94, -360, 74, -269, -33, 64, -274, 92, -375, 38, 13, -146, 95, -391, 67, -174, -65, 83, -325, 82, -336, 7, 42, -198, 95, -397, 57, -75, -83, 91, -361, 76, -288, -23, 53, -258, 87, -381, 43, 4, -127, 94, -389, 67, -210, -55, 82, -307, 85, -351, 18, 34, -184, 95, -401, 57, -101, -79, 90, -351, 79, -307, -16, 57, -240, 90, -390, 49, -20, -96, 94, -384, 69, -241, -51, 75, -290, 87, -361, 29, 27, -163, 94, -391, 59, -133, -72, 88, -341, 82, -318, -6, 53, -222, 93, -391, 50, -41, -95, 93, -362, 73, -260, -40, 71, -278, 91, -374, 36, 16, -156, 94, -390, 64, -164, -62, 82, -327, 84, -330, 3, 44, -203, 94, -393, 55, -67, -94, 95, -364, 74, -280, -28, 56, -263, 88, -382]
  out "X Output Value":i16=-32760
  out "AI2 Array back":i16[][](array[numeric])
  out "AI0 back":i16[][](array[numeric])
  out "Topography Array back":i32[][](array[numeric])
  out "Command Out":i16=-32767
  out "counter":i16
  in  "Topo Prefix 2":string
  in  "Topo Prefix 1":string
  in  "Phase Prefix 2":string
  in  "Phase Prefix 1":string
  in  "Freq Prefix 2":string
  in  "Freq Prefix 1":string
  in  "Data Directory":path=path "C:/Users/Rodolfo/Documents/LAB/2013-02-24-SPM-data"
  out "Inidicator  forth/back  Y axis":i8=1
  out "Topography Image":i32[][](graph)
  out "Trace  Topography":i32[][](graph)=[[2578410, 2578426, 2578418, 2578413, 2578392, 2578366, 2578366, 2578368, 2578377, 2578391, 2578393, 2578372, 2578349, 2578326, 2578333, 2578351, 2578378, 2578397, 2578411, 2578417, 2578388, 2578381, 2578388, 2578373, 2578375, 2578370, 2578352, 2578351, 2578349, 2578349, 2578329, 2578325, 2578341, 2578362, 2578357, 2578378, 2578397, 2578402, 2578414, 2578425, 2578437, 2578433, 2578422, 2578434, 2578407, 2578414, 2578430, 2578435, 2578443, 2578426, 2578435, 2578433, 2578438, 2578465, 2578492, 2578523, 2578533, 2578536, 2578545, 2578550, 2578565, 2578583, 2578580, 2578579, 2578566, 2578544, 2578562, 2578565, 2578572, 2578582, 2578597, 2578618, 2578638, 2578657, 2578673, 2578683, 2578690, 2578698, 2578703, 2578712, 2578717, 2578698, 2578699, 2578665, 2578667, 2578658, 2578648, 2578649, 2578647, 2578657, 2578677, 2578696, 2578724, 2578728, 2578751, 2578768, 2578763, 2578775, 2578766, 2578759, 2578740, 2578730, 2578721, 2578706, 2578697, 2578700, 2578690, 2578698, 2578720, 2578756, 2578789, 2578820, 2578841, 2578862, 2578864, 2578874, 2578873, 2578860, 2578848, 2578842, 2578831, 2578816, 2578809, 2578805, 2578792, 2578810, 2578816, 2578829, 2578835, 2578849, 2578857, 2578876, 2578897, 2578902, 2578900, 2578883, 2578874, 2578870, 2578834, 2578846, 2578835, 2578828, 2578827, 2578831, 2578846, 2578850, 2578877, 2578915, 2578931, 2578946, 2578962, 2578968, 2578971, 2578983, 2578991, 2578992, 2578978, 2578977, 2578989, 2578989, 2578998, 2579005, 2579001, 2579015, 2579038, 2579045, 2579071, 2579105, 2579131, 2579147, 2579175, 2579192, 2579208, 2579225, 2579238, 2579251, 2579258, 2579279, 2579290, 2579297, 2579301, 2579302, 2579308, 2579314, 2579324, 2579326, 2579329, 2579347, 2579375, 2579402, 2579418, 2579429, 2579443, 2579444, 2579450, 2579455, 2579465, 2579471, 2579491, 2579482, 2579492, 2579488, 2579502, 2579499, 2579515, 2579530, 2579544, 2579549, 2579534, 2579526, 2579526, 2579522, 2579545, 2579568, 2579564, 2579575, 2579577, 2579579, 2579597, 2579618, 2579650, 2579664, 2579654, 2579657, 2579668, 2579654, 2579678, 2579682, 2579677, 2579694, 2579690, 2579699, 2579706, 2579718, 2579727, 2579724, 2579747, 2579761, 2579796, 2579808, 2579832, 2579856, 2579848, 2579848, 2579835, 2579829, 2579835, 2579830, 2579830, 2579846, 2579864, 2579861, 2579869, 2579887, 2579908, 2579921, 2579930, 2579953, 2579969, 2579992, 2580010, 2580008, 2580022, 2580019, 2580020, 2580003, 2580015, 2580029, 2580023, 2580034, 2580054, 2580053, 2580054, 2580058, 2580074, 2580090, 2580115, 2580122, 2580131, 2580130, 2580151, 2580158, 2580161, 2580166, 2580163, 2580161, 2580170, 2580186, 2580198, 2580217, 2580219, 2580227, 2580251, 2580281, 2580286, 2580303, 2580310, 2580295, 2580289, 2580299, 2580294, 2580300, 2580305, 2580304, 2580312, 2580310, 2580309, 2580323, 2580346, 2580363, 2580395, 2580394, 2580403, 2580398, 2580419, 2580429, 2580447, 2580469, 2580471, 2580479, 2580494, 2580491, 2580506, 2580516, 2580508, 2580510, 2580513, 2580500, 2580520, 2580526, 2580555, 2580560, 2580568, 2580600, 2580602, 2580614, 2580613, 2580607, 2580609, 2580605, 2580607, 2580621, 2580608, 2580614, 2580618, 2580613, 2580637, 2580672, 2580683, 2580696, 2580710, 2580742, 2580750, 2580767, 2580789, 2580792, 2580809, 2580836, 2580822, 2580820, 2580823, 2580825, 2580825, 2580826, 2580821, 2580815, 2580837, 2580847, 2580852, 2580839, 2580852, 2580861, 2580879, 2580895, 2580915, 2580946, 2580960, 2580982, 2580991, 2580993, 2581001, 2581003, 2581005, 2581008, 2581024, 2581036, 2581036, 2581038, 2581029, 2581013, 2581017, 2581035, 2581057, 2581081, 2581103, 2581111, 2581118, 2581123, 2581130, 2581162, 2581186, 2581204, 2581198, 2581201, 2581200, 2581203, 2581243, 2581267, 2581284, 2581288, 2581268, 2581256, 2581248, 2581248, 2581252, 2581271, 2581281, 2581295, 2581280, 2581297, 2581312, 2581331, 2581346, 2581358, 2581373, 2581394, 2581410, 2581410, 2581413, 2581440, 2581456, 2581439, 2581449, 2581465, 2581464, 2581474, 2581469, 2581476, 2581489, 2581502, 2581513, 2581517, 2581532, 2581534, 2581538, 2581538, 2581547, 2581553, 2581554, 2581566, 2581577, 2581577, 2581582, 2581601, 2581617, 2581635, 2581639, 2581631, 2581632, 2581636, 2581643, 2581670, 2581686, 2581687, 2581695, 2581695, 2581706, 2581714, 2581736, 2581749, 2581748, 2581750, 2581767, 2581774, 2581769, 2581774, 2581775, 2581781, 2581767, 2581781, 2581797, 2581827, 2581838, 2581837, 2581859, 2581862, 2581861, 2581858, 2581883, 2581900, 2581918, 2581917, 2581928, 2581964, 2581976, 2582013, 2582004, 2582004, 2581998, 2581967, 2581970, 2581978, 2581980, 2581986, 2581999, 2581994, 2581987, 2581992, 2582001, 2582011, 2582026, 2582035], [2578296, 2578308, 2578305, 2578316, 2578335, 2578347, 2578370, 2578369, 2578388, 2578405, 2578431, 2578437, 2578452, 2578453, 2578460, 2578460, 2578464, 2578457, 2578470, 2578490, 2578495, 2578510, 2578506, 2578505, 2578515, 2578519, 2578522, 2578518, 2578542, 2578565, 2578576, 2578601, 2578619, 2578616, 2578619, 2578637, 2578652, 2578656, 2578632, 2578634, 2578629, 2578619, 2578631, 2578637, 2578641, 2578630, 2578619, 2578625, 2578635, 2578669, 2578688, 2578694, 2578705, 2578707, 2578722, 2578736, 2578744, 2578751, 2578737, 2578742, 2578746, 2578747, 2578752, 2578772, 2578785, 2578786, 2578780, 2578783, 2578788, 2578782, 2578795, 2578813, 2578815, 2578839, 2578839, 2578835, 2578838, 2578859, 2578874, 2578893, 2578912, 2578921, 2578930, 2578939, 2578936, 2578943, 2578966, 2579002, 2579023, 2579033, 2579051, 2579059, 2579052, 2579050, 2579069, 2579070, 2579077, 2579087, 2579091, 2579101, 2579093, 2579113, 2579120, 2579126, 2579137, 2579149, 2579157, 2579164, 2579175, 2579185, 2579182, 2579162, 2579155, 2579132, 2579145, 2579158, 2579148, 2579154, 2579154, 2579162, 2579155, 2579148, 2579156, 2579175, 2579178, 2579202, 2579216, 2579217, 2579223, 2579234, 2579241, 2579258, 2579266, 2579275, 2579255, 2579263, 2579267, 2579277, 2579289, 2579312, 2579319, 2579329, 2579321, 2579332, 2579330, 2579330, 2579337, 2579345, 2579367, 2579372, 2579355, 2579367, 2579379, 2579386, 2579388, 2579382, 2579391, 2579400, 2579391, 2579388, 2579382, 2579386, 2579387, 2579403, 2579419, 2579422, 2579433, 2579422, 2579435, 2579469, 2579492, 2579511, 2579549, 2579578, 2579577, 2579597, 2579618, 2579641, 2579655, 2579675, 2579700, 2579717, 2579740, 2579760, 2579778, 2579796, 2579813, 2579813, 2579814, 2579833, 2579856, 2579878, 2579891, 2579891, 2579891, 2579881, 2579882, 2579890, 2579889, 2579896, 2579901, 2579922, 2579935, 2579933, 2579957, 2579965, 2579977, 2579989, 2579993, 2580012, 2580009, 2580017, 2580022, 2580034, 2580035, 2580036, 2580032, 2580042, 2580060, 2580072, 2580084, 2580090, 2580110, 2580117, 2580136, 2580128, 2580132, 2580151, 2580155, 2580169, 2580149, 2580149, 2580146, 2580148, 2580151, 2580151, 2580153, 2580159, 2580185, 2580190, 2580184, 2580191, 2580205, 2580221, 2580250, 2580262, 2580271, 2580278, 2580298, 2580298, 2580308, 2580317, 2580322, 2580349, 2580352, 2580373, 2580384, 2580392, 2580393, 2580392, 2580407, 2580423, 2580418, 2580413, 2580418, 2580411, 2580419, 2580413, 2580412, 2580419, 2580422, 2580439, 2580436, 2580447, 2580467, 2580480, 2580489, 2580503, 2580517, 2580534, 2580545, 2580561, 2580570, 2580563, 2580570, 2580580, 2580577, 2580591, 2580588, 2580583, 2580602, 2580608, 2580606, 2580620, 2580612, 2580618, 2580624, 2580644, 2580674, 2580675, 2580699, 2580705, 2580707, 2580715, 2580726, 2580722, 2580719, 2580716, 2580725, 2580725, 2580753, 2580771, 2580776, 2580773, 2580780, 2580794, 2580792, 2580802, 2580816, 2580816, 2580816, 2580842, 2580858, 2580865, 2580879, 2580883, 2580899, 2580907, 2580900, 2580905, 2580919, 2580922, 2580936, 2580939, 2580962, 2580980, 2581011, 2581018, 2581015, 2581021, 2581036, 2581049, 2581058, 2581069, 2581072, 2581069, 2581064, 2581075, 2581068, 2581068, 2581089, 2581086, 2581105, 2581112, 2581118, 2581137, 2581155, 2581174, 2581197, 2581209, 2581211, 2581230, 2581248, 2581254, 2581273, 2581267, 2581254, 2581242, 2581240, 2581248, 2581253, 2581274, 2581272, 2581265, 2581276, 2581272, 2581284, 2581291, 2581304, 2581331, 2581341, 2581347, 2581342, 2581335, 2581336, 2581347, 2581351, 2581356, 2581363, 2581380, 2581384, 2581404, 2581429, 2581439, 2581469, 2581482, 2581483, 2581486, 2581478, 2581477, 2581456, 2581443, 2581434, 2581422, 2581429, 2581426, 2581434, 2581446, 2581449, 2581449, 2581492, 2581511, 2581525, 2581550, 2581566, 2581570, 2581578, 2581591, 2581604, 2581600, 2581595, 2581606, 2581615, 2581618, 2581613, 2581608, 2581626, 2581622, 2581629, 2581654, 2581686, 2581714, 2581736, 2581761, 2581764, 2581759, 2581760, 2581760, 2581755, 2581769, 2581771, 2581756, 2581755, 2581751, 2581759, 2581755, 2581750, 2581757, 2581753, 2581758, 2581779, 2581804, 2581820, 2581846, 2581850, 2581846, 2581845, 2581849, 2581836, 2581834, 2581830, 2581814, 2581845, 2581859, 2581872, 2581895, 2581894, 2581902, 2581916, 2581939, 2581949, 2581966, 2581976, 2581997, 2582004, 2582021, 2582021, 2582019, 2582019, 2582011, 2581998, 2582005, 2581989, 2581990, 2581994, 2581994, 2582011, 2581993, 2581993, 2581988, 2581985, 2581987, 2581990, 2582004, 2581993, 2582006, 2582016, 2582049, 2582067, 2582092, 2582101, 2582097, 2582091, 2582083, 2582079, 2582069, 2582071, 2582056, 2582049, 2582044, 2582033, 2582029]]
  out "Topography Array":i32[][](array[numeric])
  in  "New Image":bool
  out "error out 2":errorcluster
  out "error out":errorcluster
  out "Bottom Sensor Phase  Image":i16[][](graph)
  out "Trace Bottom Sensor Phase":i16[][](graph)=[[80, -305, 87, -353, 20, 35, -176, 95, -394, 58, -111, -77, 89, -347, 82, -308, -11, 55, -233, 92, -393, 51, -27, -96, 94, -378, 71, -240, -45, 74, -282, 87, -365, 33, 25, -159, 95, -391, 61, -146, -67, 87, -335, 80, -324, -3, 51, -215, 94, -395, 51, -49, -95, 93, -363, 76, -273, -34, 62, -277, 93, -374, 38, 13, -137, 95, -389, 65, -183, -59, 82, -320, 82, -340, 9, 40, -192, 95, -401, 55, -82, -87, 91, -362, 77, -292, -24, 57, -250, 87, -385, 45, -5, -123, 96, -392, 66, -221, -53, 80, -304, 86, -356, 21, 30, -178, 94, -395, 57, -113, -78, 87, -346, 78, -308, -12, 55, -234, 89, -392, 50, -26, -96, 94, -379, 72, -236, -43, 71, -286, 87, -369, 31, 22, -160, 94, -395, 62, -149, -69, 85, -341, 82, -328, -2, 46, -213, 92, -395, 52, -56, -98, 92, -363, 76, -269, -32, 64, -272, 91, -377, 38, 15, -145, 93, -390, 63, -181, -61, 82, -321, 82, -341, 10, 41, -197, 92, -398, 56, -80, -84, 91, -358, 77, -288, -24, 53, -254, 87, -385, 45, -4, -126, 95, -390, 67, -217, -54, 82, -304, 86, -353, 20, 33, -175, 95, -397, 58, -110, -74, 89, -350, 79, -311, -13, 54, -234, 92, -391, 48, -27, -92, 91, -378, 72, -243, -43, 72, -291, 87, -366, 30, 23, -163, 96, -390, 60, -146, -68, 87, -336, 82, -324, 0, 51, -216, 92, -396, 53, -51, -95, 94, -361, 75, -272, -33, 62, -268, 90, -378, 36, 13, -143, 94, -389, 64, -181, -63, 81, -323, 86, -343, 9, 41, -197, 93, -390, 57, -80, -87, 91, -358, 79, -295, -23, 55, -252, 86, -386, 43, -9, -120, 97, -390, 67, -221, -51, 79, -304, 87, -355, 22, 33, -178, 93, -400, 59, -111, -79, 90, -348, 78, -310, -11, 55, -232, 92, -391, 46, -26, -92, 95, -375, 69, -233, -45, 73, -285, 90, -366, 32, 26, -159, 95, -395, 62, -148, -71, 85, -338, 84, -325, -2, 49, -215, 93, -398, 54, -52, -93, 93, -360, 72, -276, -33, 62, -271, 91, -378, 42, 14, -142, 96, -389, 67, -185, -62, 81, -323, 83, -339, 9, 39, -195, 93, -396, 55, -79, -87, 90, -365, 78, -294, -25, 56, -251, 86, -384, 45, -7, -117, 93, -388, 68, -216, -52, 81, -303, 84, -354, 22, 33, -172, 93, -394, 60, -118, -77, 89, -344, 80, -308, -11, 53, -231, 90, -391, 50, -29, -88, 95, -375, 70, -254, -47, 74, -281, 91, -371, 31, 25, -156, 97, -393, 63, -149, -69, 86, -331, 81, -327, 0, 49, -214, 92, -396, 55, -54, -94, 91, -361, 75, -272, -31, 59, -272, 91, -377, 42, 12, -140, 96, -388, 66, -189, -61, 83, -314, 83, -342, 11, 40, -194, 92, -397, 55, -84, -81, 92, -358, 77, -293, -20, 55, -252, 87, -387, 47, -6, -116, 96, -389, 68, -225, -52, 78, -302, 86, -356, 23, 34, -169, 95, -396, 60, -120, -76, 87, -347, 80, -310, -7], [-342, 80, -313, 82, -58, -196, 66, -389, 96, -132, 5, 45, -377, 90, -264, 59, -27, -280, -311, 76, -349, 88, -76, -113, 57, -396, 94, -175, 34, 18, -351, 85, -305, 82, -53, -219, 69, -386, 94, -123, -5, 44, -386, 86, -254, 53, -21, -292, 76, -361, 89, -83, -83, 55, -399, 95, -192, 39, 11, -342, 83, -319, 80, -54, -185, 68, -389, 93, -136, 11, 40, -377, 89, -270, 62, -31, -274, 76, -359, 92, -94, -52, 54, -396, 92, -213, 46, 3, -328, 81, -333, 85, -69, -151, 64, -393, 94, -159, 19, 31, -371, 89, -288, 71, -43, -249, 70, -370, 95, -88, -28, 51, -391, 91, -231, 55, -7, -307, 80, -347, 88, -74, -114, 60, -391, 97, -175, 35, 22, -355, 87, -302, 81, -53, -226, 68, -387, 94, -110, -6, 46, -385, 86, -249, 54, -20, -294, 77, -356, 90, -85, -84, 56, -394, 95, -191, 39, 11, -340, 83, -316, 80, -60, -187, 64, -388, 96, -138, 10, 39, -378, 91, -270, 61, -34, -270, 72, -357, 92, -92, -56, 52, -396, 92, -212, 50, 2, -327, 84, -331, 87, -69, -155, 61, -393, 95, -154, 25, 36, -367, 89, -291, 72, -42, -252, 71, -371, 93, -93, -29, 51, -393, 94, -231, 53, -10, -313, 80, -344, 88, -75, -111, 60, -394, 95, -166, 32, 23, -355, 86, -301, 79, -50, -222, 69, -388, 95, -116, -7, 46, -384, 87, -248, 56, -21, -294, 77, -357, 93, -82, -88, 58, -391, 93, -193, 40, 11, -343, 83, -316, 84, -59, -191, 67, -386, 96, -137, 11, 40, -379, 92, -269, 59, -31, -275, 73, -359, 93, -93, -53, 52, -397, 92, -212, 48, -1, -326, 82, -331, 86, -65, -152, 60, -390, 94, -158, 23, 36, -366, 90, -282, 72, -42, -250, 73, -369, 93, -92, -28, 49, -393, 91, -228, 55, -9, -312, 79, -341, 88, -75, -115, 58, -394, 93, -174, 32, 22, -352, 86, -302, 78, -49, -219, 67, -387, 93, -115, -5, 45, -386, 89, -245, 54, -16, -288, 79, -355, 91, -85, -83, 55, -397, 97, -191, 40, 12, -341, 83, -321, 81, -59, -191, 64, -387, 94, -131, 10, 40, -377, 92, -266, 59, -29, -274, 75, -360, 91, -87, -63, 51, -395, 93, -211, 47, 1, -326, 84, -331, 85, -67, -155, 62, -390, 96, -157, 21, 32, -369, 88, -285, 72, -40, -254, 70, -368, 95, -91, -29, 51, -399, 92, -231, 50, -10, -312, 79, -346, 87, -73, -119, 58, -396, 95, -172, 32, 24, -361, 86, -297, 79, -50, -227, 67, -388, 94, -117, -11, 49, -385, 87, -249, 53, -16, -295, 77, -355, 89, -78, -83, 56, -397, 94, -193, 41, 12, -344, 86, -315, 82, -63, -189, 65, -388, 95, -131, 11, 39, -379, 88, -269, 57, -28, -275, 76, -361, 90, -90, -55, 55, -393, 93, -210, 48, 3, -327, 82, -330, 86, -67, -154, 62, -392, 94, -156, 23, 35, -363, 88, -282, 72, -42, -251, 70, -372, 95, -89, -30, 50, -393, 92, -232, 55]]
  out "Trace Frequency":i16[][](graph)=[[45, -178, 33, -89, -19, 26, -131, 45, -151, 10, 0, -80, 44, -182, 29, -62, -45, 30, -156, 41, -125, 2, 16, -83, 46, -175, 18, -40, -65, 39, -175, 36, -95, -12, 23, -123, 47, -156, 14, -10, -75, 47, -182, 30, -70, -36, 27, -149, 43, -136, 5, 12, -87, 48, -172, 23, -48, -58, 32, -170, 42, -107, -6, 23, -113, 48, -164, 14, -20, -71, 42, -181, 30, -79, -29, 25, -143, 45, -145, 8, 6, -84, 46, -182, 26, -57, -52, 25, -162, 34, -116, 1, 22, -104, 48, -174, 17, -30, -69, 45, -178, 33, -87, -21, 25, -133, 45, -151, 10, 0, -80, 46, -182, 27, -62, -42, 28, -156, 41, -125, 4, 16, -82, 49, -174, 23, -32, -64, 39, -175, 35, -99, -12, 23, -126, 45, -156, 14, -9, -76, 47, -181, 31, -69, -39, 26, -149, 43, -139, 8, 13, -85, 49, -169, 23, -46, -57, 30, -172, 42, -108, -6, 21, -118, 46, -165, 15, -19, -72, 43, -181, 32, -79, -29, 25, -143, 43, -145, 9, 7, -81, 47, -180, 29, -54, -53, 25, -164, 35, -116, -3, 23, -105, 49, -174, 18, -29, -69, 47, -177, 36, -86, -23, 26, -130, 44, -150, 10, 0, -77, 46, -179, 29, -60, -44, 30, -158, 38, -127, 3, 18, -82, 49, -175, 22, -32, -64, 42, -173, 37, -96, -13, 25, -127, 47, -156, 13, -8, -75, 46, -181, 33, -68, -37, 28, -150, 41, -136, 5, 12, -88, 48, -171, 24, -47, -55, 32, -171, 41, -107, -7, 24, -119, 45, -165, 16, -18, -74, 43, -182, 31, -79, -30, 28, -139, 43, -146, 8, 6, -83, 46, -179, 27, -52, -49, 27, -162, 34, -118, -1, 21, -102, 45, -174, 18, -31, -69, 47, -176, 36, -86, -20, 27, -132, 46, -152, 9, -1, -79, 48, -180, 27, -62, -42, 29, -155, 39, -126, 4, 16, -83, 48, -174, 22, -35, -65, 43, -173, 37, -96, -12, 23, -124, 46, -160, 12, -7, -74, 44, -181, 32, -67, -37, 29, -146, 42, -136, 4, 12, -87, 47, -172, 24, -46, -56, 31, -168, 42, -106, -6, 22, -113, 48, -164, 14, -20, -71, 43, -178, 31, -78, -28, 28, -140, 44, -143, 9, 7, -83, 48, -181, 27, -56, -50, 27, -163, 35, -116, 0, 20, -104, 47, -174, 19, -30, -67, 46, -176, 33, -87, -18, 27, -130, 46, -150, 11, 0, -78, 46, -182, 27, -63, -42, 30, -158, 42, -127, 3, 16, -81, 49, -174, 19, -41, -65, 40, -173, 35, -99, -12, 25, -126, 45, -159, 12, -9, -76, 46, -183, 33, -72, -36, 27, -149, 42, -137, 5, 13, -86, 48, -171, 23, -51, -57, 28, -169, 41, -108, -5, 24, -114, 48, -165, 17, -21, -73, 42, -180, 31, -78, -30, 26, -142, 43, -145, 9, 5, -81, 49, -178, 25, -57, -51, 27, -164, 36, -120, 0, 19, -100, 49, -175, 18, -32, -71, 45, -178, 32, -89, -19, 26, -129, 47, -149, 12, -2, -79, 47, -180, 27, -62, -44], [-82, 32, -177, 42, -72, -22, 15, -169, 47, -110, 22, -6, -112, 42, -169, 27, -55, -49, -62, 28, -182, 45, -77, 0, 10, -153, 46, -133, 26, -22, -87, 36, -177, 47, -66, -30, 17, -173, 46, -103, 19, -1, -118, 34, -165, 26, -51, -53, 25, -179, 46, -81, 6, 9, -146, 43, -140, 24, -29, -80, 32, -181, 43, -71, -21, 17, -165, 46, -115, 24, -5, -108, 39, -168, 30, -56, -48, 23, -174, 47, -87, 12, 6, -138, 42, -149, 28, -37, -70, 32, -180, 45, -73, -9, 15, -160, 46, -126, 24, -13, -98, 40, -174, 40, -65, -39, 21, -170, 48, -82, 16, 3, -128, 40, -158, 30, -43, -62, 29, -179, 46, -77, 1, 12, -151, 44, -129, 24, -18, -90, 34, -177, 47, -67, -30, 18, -174, 46, -100, 21, 1, -118, 34, -162, 24, -51, -56, 27, -179, 49, -81, 6, 8, -146, 42, -141, 26, -28, -80, 33, -181, 40, -73, -20, 16, -165, 48, -117, 23, -8, -110, 42, -172, 27, -57, -49, 22, -173, 48, -86, 13, 7, -137, 43, -146, 27, -39, -71, 29, -182, 46, -75, -10, 12, -157, 45, -126, 24, -11, -100, 34, -174, 39, -63, -44, 20, -170, 50, -80, 17, 6, -131, 42, -159, 27, -43, -65, 27, -181, 45, -79, -2, 9, -153, 46, -128, 23, -18, -88, 34, -177, 45, -68, -31, 17, -176, 50, -99, 22, 1, -118, 35, -161, 29, -50, -54, 27, -182, 47, -84, 6, 9, -146, 44, -140, 26, -29, -80, 33, -179, 42, -71, -23, 18, -163, 47, -111, 23, -3, -110, 42, -168, 29, -55, -49, 22, -175, 46, -87, 12, 6, -137, 44, -149, 27, -35, -69, 31, -183, 44, -75, -11, 13, -161, 46, -123, 25, -12, -98, 38, -172, 39, -63, -40, 21, -174, 48, -84, 17, 5, -130, 40, -154, 29, -44, -64, 28, -182, 45, -79, 0, 10, -153, 46, -129, 27, -17, -87, 34, -175, 46, -68, -31, 19, -175, 47, -101, 21, 1, -117, 36, -161, 28, -48, -55, 26, -181, 47, -83, 5, 8, -148, 45, -140, 26, -26, -78, 32, -176, 43, -71, -22, 17, -168, 47, -110, 24, -5, -109, 41, -169, 26, -54, -49, 25, -173, 48, -85, 10, 4, -137, 42, -146, 27, -32, -69, 32, -180, 45, -74, -10, 13, -160, 45, -128, 22, -12, -100, 38, -172, 42, -62, -41, 21, -170, 48, -81, 16, 5, -131, 41, -155, 29, -41, -64, 29, -181, 48, -77, -1, 10, -152, 45, -132, 24, -19, -90, 36, -175, 45, -67, -30, 20, -176, 48, -99, 18, 1, -119, 36, -161, 27, -51, -56, 27, -180, 48, -81, 6, 9, -147, 43, -139, 24, -28, -81, 33, -179, 43, -71, -23, 16, -166, 46, -108, 22, -4, -111, 41, -168, 27, -57, -50, 25, -174, 49, -86, 9, 4, -137, 44, -147, 26, -36, -72, 32, -181, 47, -75, -10, 14, -160, 46, -125, 23, -10, -99, 39, -174, 39, -64, -41, 22, -171, 49, -81, 16, 3, -128, 43, -158, 31]]
  out "Frequency Shift Image":i16[][](graph)
  out "AI0 Array":i16[][](array[numeric])
  out "AI2 Array":i16[][](array[numeric])
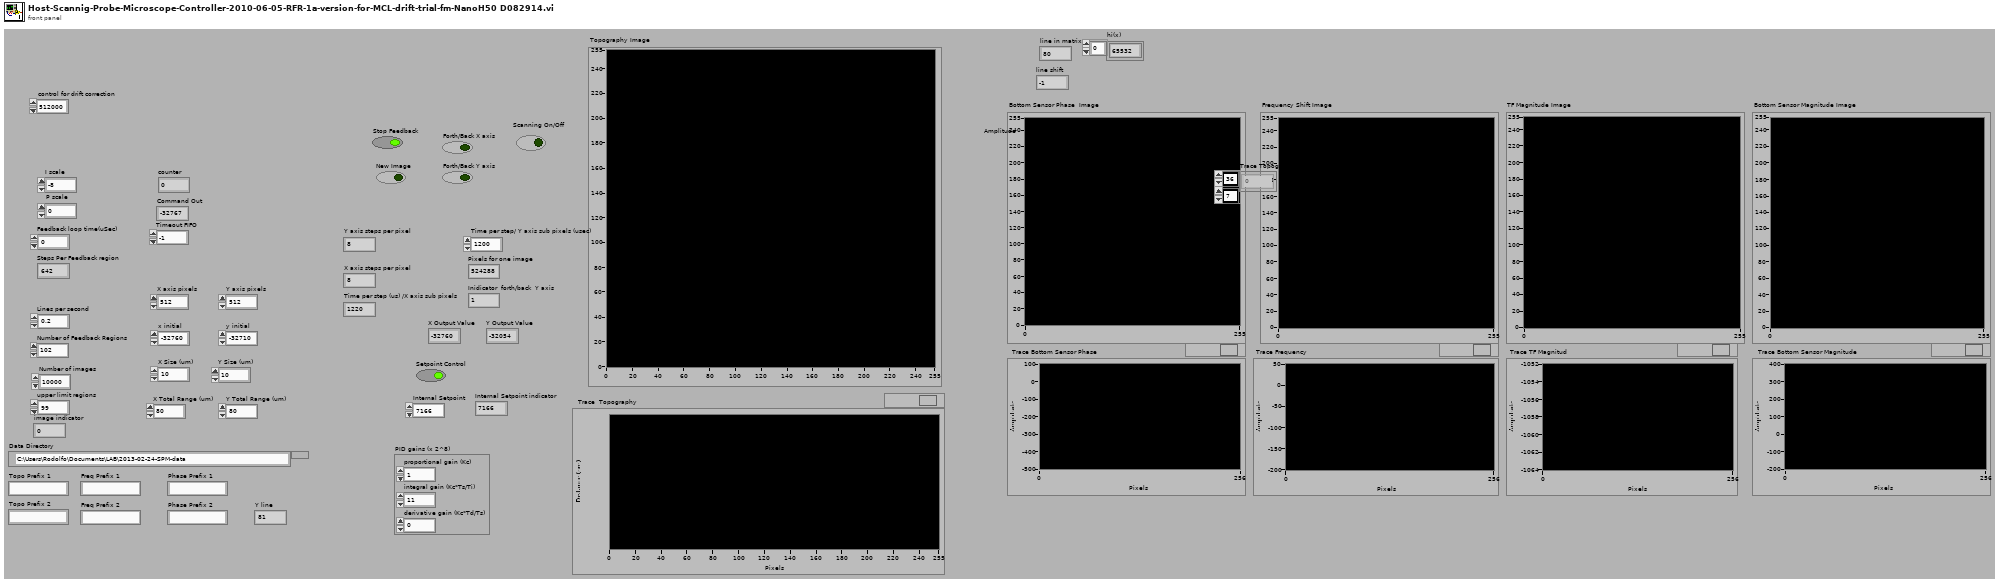
[diagram p1: front panel]
types:
  T1 = cluster{"proportional gain (Kc)":i16, "integral gain (Kc*Ts/Ti)":i16, "derivative gain (Kc*Td/Ts)":i16}
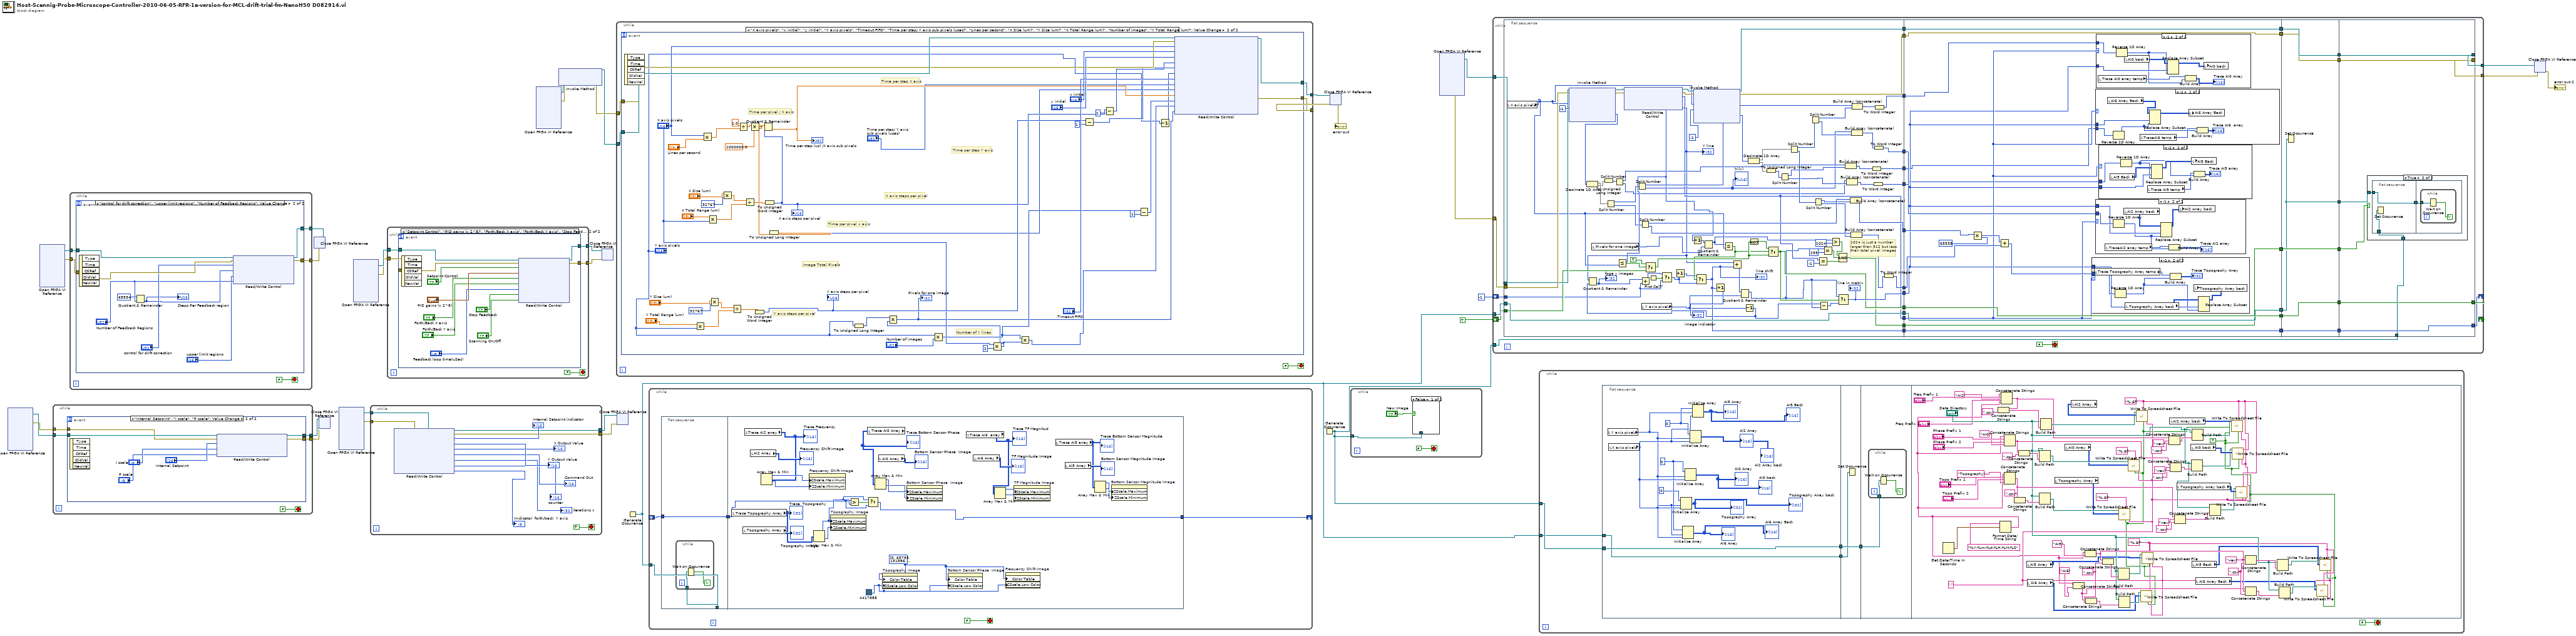
[diagram p0: block diagram]
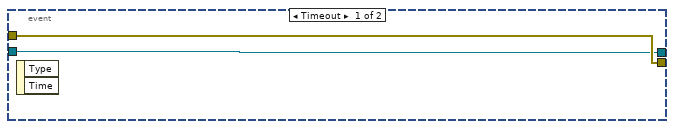
[diagram p2: hidden frame]
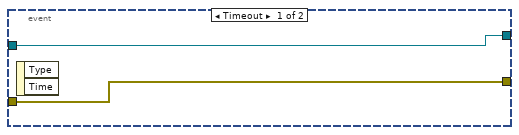
[diagram p3: hidden frame]
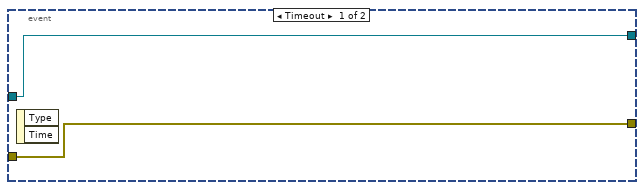
[diagram p4: hidden frame]
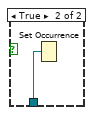
[diagram p5: hidden frame]
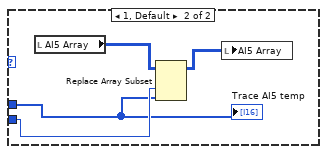
[diagram p6: hidden frame]
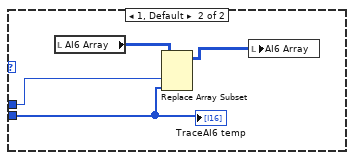
[diagram p7: hidden frame]
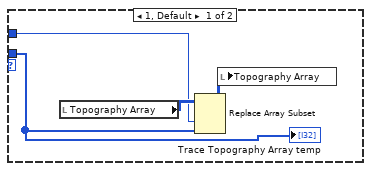
[diagram p8: hidden frame]
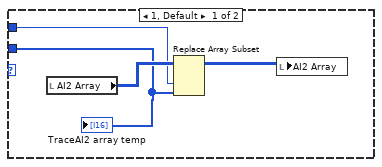
[diagram p9: hidden frame]
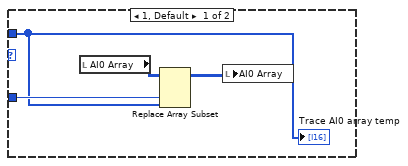
[diagram p10: hidden frame]
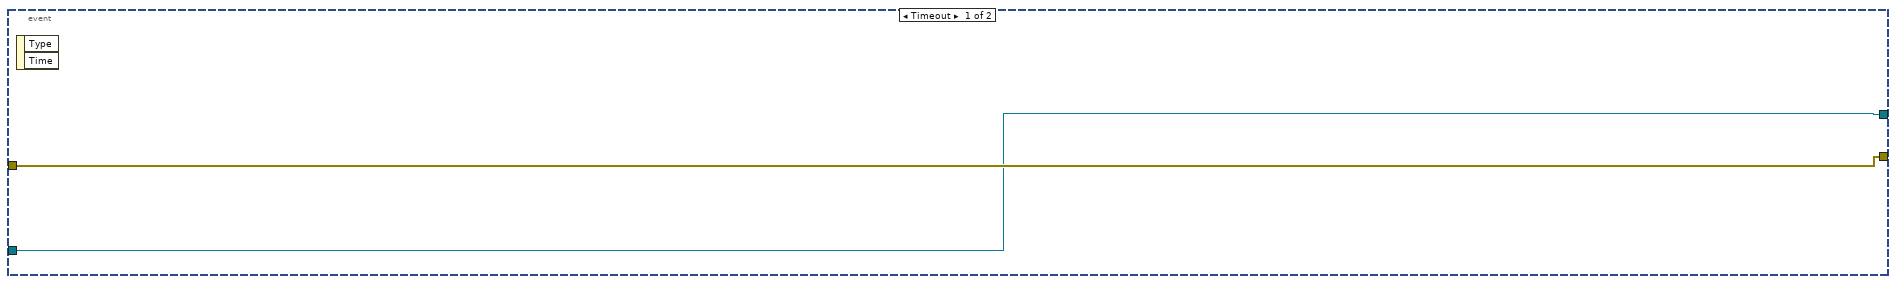
[diagram p12: hidden frame]
diagram:
  n1 = xnode "Open FPGA VI Reference"() -> ("FPGA VI Reference Out"=w12:refnum<k20>, "error out"=w11:errorcluster)  [unwired: 2 in]
  n2 = xnode "Open FPGA VI Reference"() -> ("FPGA VI Reference Out"=w16:refnum<k20>, "error out"=w15:errorcluster)  [unwired: 2 in]
  n3 = while {
    tunnel: w12 -> [w37]
    tunnel: w11 -> [w36]
    tunnel: [w34] -> w6
    tunnel: [w33] -> w5
    stop <- FALSE stop-if-true
    n4 = event shown="[1] \"Internal Setpoint\", \"I scale\", \"P scale\": Value Change" {
      selector: _ -> [_ _]
      dyn-events: _ -> [_ _]
      timeout: _ -> [_ _]
      tunnel: w37 -> [w38 w46]
      tunnel: w36 -> [w39 w45]
      tunnel: [w38 w41] -> w34
      tunnel: [w39 w40] -> w33
      event Timeout {
        n5 = event-data() -> ()  [unwired: 1 in, 2 out]
      }
      event "Internal Setpoint", "I scale", "P scale": Value Change {
        n6 = event-data() -> ()  [unwired: 1 in, 5 out]
        n7 = xnode "Read/Write Control"("FPGA VI Reference In"=w46, "error in"=w45, "Internal Setpoint External Control"="Internal Setpoint", "I scale"="I scale", "P scale"="P scale") -> ("FPGA VI Reference Out"=w41:refnum<k20>, "error out"=w40:errorcluster)
      }
    }
  }
  n8 = while {
    tunnel: w16 -> [w51]
    tunnel: w15 -> [w50]
    tunnel: [w48] -> w2
    tunnel: [w47] -> w1
    stop <- FALSE stop-if-true
    n9 = event shown="[1] \" control for drift correction\", \"upper limit regions\", \"Number of Feedback Regions\": Value Change" {
      selector: _ -> [_ _]
      dyn-events: _ -> [_ _]
      timeout: _ -> [_ _]
      tunnel: w51 -> [w53 w62]
      tunnel: w50 -> [w52 w61]
      tunnel: [w53 w55] -> w48
      tunnel: [w52 w54] -> w47
      event Timeout {
        n10 = event-data() -> ()  [unwired: 1 in, 2 out]
      }
      event "control for drift correction", "upper limit regions", "Number of Feedback Regions": Value Change {
        n11 = event-data() -> ()  [unwired: 1 in, 5 out]
        n12 = Quotient & Remainder(x=u32 65534, y="Number of Feedback Regions") -> (floor(x/y)=w57:u32)  [unwired: 1 out]
        "Steps Per Feedback region" <- w57
        n13 = xnode "Read/Write Control"("FPGA VI Reference In"=w62, "error in"=w61, "drift temporal control"="control for drift correction", "Steps per Feedback Region"=w57, "provisional limit"="upper limit regions", "shift-divisions (always >=2)"="Number of Feedback Regions") -> ("FPGA VI Reference Out"=w55:refnum<k20>, "error out"=w54:errorcluster)
      }
    }
  }
  n14 = xnode "Close FPGA VI Reference"("FPGA VI Reference In"=w2, "error in"=w1) -> ()  [unwired: 1 out]
  n15 = xnode "Close FPGA VI Reference"("FPGA VI Reference In"=w6, "error in"=w5) -> ()  [unwired: 1 out]
  n16 = xnode "Open FPGA VI Reference"() -> ("FPGA VI Reference Out"=w10:refnum<k20>, "error out"=w9:errorcluster)  [unwired: 2 in]
  n17 = xnode "Open FPGA VI Reference"() -> ("FPGA VI Reference Out"=w14:refnum<k20>, "error out"=w13:errorcluster)  [unwired: 2 in]
  n18 = while {
    tunnel: w10 -> [w74]
    tunnel: w9 -> [w73]
    tunnel: [w64] -> w8
    tunnel: [w63] -> w7
    stop <- FALSE stop-if-true
    n19 = xnode "Read/Write Control"("FPGA VI Reference In"=w74, "error in"=w73) -> ("FPGA VI Reference Out"=w64:refnum<k20>, "error out"=w63:errorcluster, "Internal Setpoint"=→"Internal Setpoint indicator":i16, "X Output Value"=→"X Output Value":i16, "Y Output Value"=→"Y Output Value":i16, "Command Out"=→"Command Out":i16, "iterations x"=→"iterations x":i32, "Counter Data"=→"counter":i8, "Inidicator  forth/back  Y axis"=→"Inidicator  forth/back  Y axis":i8)
  }
  n20 = while {
    tunnel: w14 -> [w79]
    tunnel: w13 -> [w78]
    tunnel: [w76] -> w4
    tunnel: [w75] -> w3
    stop <- FALSE stop-if-true
    n21 = event shown="[1] \"Setpoint Control\", \"PID gains (x 2^8)\", \"Forth/Back X axis\", \"Forth/Back Y axis\", \"Stop Feedback\", \"Scanning On/Off\", \"Feedback loop time(uSec)\": Value Change" {
      selector: _ -> [_ _]
      dyn-events: _ -> [_ _]
      timeout: _ -> [_ _]
      tunnel: w79 -> [w81 w92]
      tunnel: w78 -> [w80 w91]
      tunnel: [w81 w83] -> w76
      tunnel: [w80 w82] -> w75
      event Timeout {
        n22 = event-data() -> ()  [unwired: 1 in, 2 out]
      }
      event "Setpoint Control", "PID gains (x 2^8)", "Forth/Back X axis", "Forth/Back Y axis", "Stop Feedback", "Scanning On/Off", "Feedback loop time(uSec)": Value Change {
        n23 = event-data() -> ()  [unwired: 1 in, 5 out]
        n24 = xnode "Read/Write Control"("FPGA VI Reference In"=w92, "error in"=w91, "Setpoint Control"="Setpoint Control", "PID gains (x 2^8)"="PID gains (x 2^8)", "Forth/Back X axis"="Forth/Back X axis", "Forth/Back Y axis"="Forth/Back Y axis", "Count(uSec)"="Feedback loop time(uSec)", "Stop Feedback Control"="Stop Feedback", "Scanning On/Off"="Scanning On/Off") -> ("FPGA VI Reference Out"=w83:refnum<k20>, "error out"=w82:errorcluster)
      }
    }
  }
  n25 = xnode "Open FPGA VI Reference"() -> ("FPGA VI Reference Out"=w22:refnum<k20>, "error out"=w21:errorcluster)  [unwired: 2 in]
  n26 = xnode "Invoke Method"("FPGA VI Reference In"=w22, "error in"=w21) -> ("FPGA VI Reference Out"=w19:refnum<k20>, "error out"=w20:errorcluster)  [unwired: 1 in]
  n27 = xnode "Close FPGA VI Reference"("FPGA VI Reference In"=w4, "error in"=w3) -> ()  [unwired: 1 out]
  n28 = while {
    tunnel: w20 -> [w94]
    tunnel: w19 -> [w97]
    tunnel: [w96] -> w31
    tunnel: [w95] -> w30
    stop <- FALSE stop-if-true
    n29 = event shown="[1] \"X axis pixels\", \"x initial\", \"y initial\", \"Y axis pixels\", \"Timeout FIFO\", \"Time per step/ Y axis sub pixels (usec)\", \"Lines per second\", \"X Size (um)\", \"Y Size (um)\", \"X Total Range (um)\", \"Number of images\", \"Y Total Range (um)\": Value Change" {
      selector: _ -> [_ _]
      dyn-events: _ -> [_ _]
      timeout: _ -> [_ _]
      tunnel: w97 -> [w98 w128]
      tunnel: [w98 w127] -> w96
      tunnel: [w99 w126] -> w95
      tunnel: w94 -> [w99 w125]
      event Timeout {
        n30 = event-data() -> ()  [unwired: 1 in, 2 out]
      }
      event "X axis pixels", "x initial", "y initial", "Y axis pixels", "Timeout FIFO", "Time per step/ Y axis sub pixels (usec)", "Lines per second", "X Size (um)", "Y Size (um)", "X Total Range (um)", "Number of images", "Y Total Range (um)": Value Change {
        # "Number of Y lines"
        # "Time per step Y axis"
        # "Time per step X axis"
        # "Time per pixel x axis"
        # "Image Total Pixels"
        # "Y axis steps per pixel"
        # "Time per pixel / X axis"
        # "X axis steps per pixel"
        n31 = event-data() -> ()  [unwired: 1 in, 5 out]
        n32 = Multiply(x="Y Total Range (um)", y="Y axis pixels") -> (x*y=w133:dbl)
        n33 = Multiply(x="X axis pixels", y="Lines per second") -> (x*y=w145:dbl)
        n34 = Multiply(x="X Total Range (um)", y="X axis pixels") -> (x*y=w139:dbl)
        n35 = Multiply(x="Y Size (um)", y=i16 32767) -> (x*y=w135:dbl)
        n36 = Multiply(x="X Size (um)", y=i16 32767) -> (x*y=w141:dbl)
        n37 = Divide(x=w135, y=w133) -> (x/y=w132:dbl)
        n38 = Divide(x=1.0, y=w145) -> (x/y=w124:dbl)
        n39 = Divide(x=w141, y=w139) -> (x/y=w122:dbl)
        n40 = Multiply(x=w124, y=1000000.0) -> (x*y=w121:dbl)
        n41 = To Unsigned Word Integer(number=w132) -> (unsigned 16bit integer=w117:u16)
        "Y axis steps per pixel" <- w117
        n42 = To Unsigned Word Integer(number=w122) -> (unsigned 16bit integer=w120:u16)
        "X axis steps per pixel" <- w120
        n43 = Quotient & Remainder(x=w121, y=w120) -> (floor(x/y)=w114:dbl)  [unwired: 1 out]
        "Time per step (us) /X axis sub pixels" <- w114
        n44 = To Unsigned Long Integer(number=w121) -> (unsigned 32bit integer=w113:u32)
        n45 = To Unsigned Long Integer(number="Y axis pixels") -> (unsigned 32bit integer=w101:u32)
        n46 = Multiply(x="Y axis pixels", y="Number of images") -> (x*y=w108:u32)
        n47 = Multiply(x="X axis pixels", y=u16 2) -> (x*y=w104:u16)
        n48 = Multiply(x=w101, y=w104) -> (x*y=w103:u32)
        "Pixels for one image" <- w103
        n49 = Multiply(x=w108, y=w104) -> (x*y=w100:u32)
        n50 = Subtract(x=w117, y=u16 1) -> (x-y=w115:u16)
        n51 = Subtract(x=w120, y=u16 1) -> (x-y=w118:u16)
        n52 = Subtract(x=w108, y=u32 1) -> (x-y=w109:u32)
        n53 = Decrement(x="Y axis pixels") -> (x-1=w105:u16)
        n54 = xnode "Read/Write Control"("FPGA VI Reference In"=w128, "error in"=w125, "X axis pixels"="X axis pixels", "x initial"="x initial", "y initial"="y initial", "X steps per pixel"=w118, "Y steps per pixel"=w115, "Y axis pixels"=w105, "Timeout FIFO"="Timeout FIFO", "Time per step/ Y axis sub pixel (uSec)"="Time per step/ Y axis sub pixels (usec)", "Time per image pixel/ X axis pixel (uSec)"=w113, "Time per step/ X axis sub pixel (uSec)"=w114, "Y Number of Lines"=w109, "Image Total Pixels"=w100, "Pixels in one image"=w103) -> ("FPGA VI Reference Out"=w127:refnum<k20>, "error out"=w126:errorcluster)
      }
    }
  }
  n55 = xnode "Close FPGA VI Reference"("FPGA VI Reference In"=w8, "error in"=w7) -> ()  [unwired: 1 out]
  n56 = Generate Occurrence() -> (w24:refnum<k4>)
  n57 = while {
    tunnel: w24 -> [w149]
    shift-right: [w148] -> _
    shift-left: _ -> [w146]
    stop <- FALSE stop-if-true
    n58 = flat-sequence {
      tunnel: w149 -> [w152]
      tunnel: [w151] -> w147
      tunnel: w146 -> [w151]
      tunnel: [w157] -> w148
      tunnel: w147 -> [w155]
      frame #0 {
        n59 = while {
          tunnel: w152 -> [w153]
          stop <- w154 continue-if-true
          n60 = Wait on Occurrence(2:w153) -> (0:w154:bool)  [unwired: 2 in]
        }
      }
      frame #1 {
        w169 = u32[] [0, 65793, 131586, 197379, 263172, 328965, 394758, 460551, 526344, 592137, 657930, 723723, 789516, 855309, 921102, 986895, 1052688, 1118481, 1184274, 1250067, 1315860, 1381653, 1447446, 1513239, 1579032, 1644825, 1710618, 1776411, 1842204, 1907997, 1973790, 2039583, 2105376, 2171169, 2236962, 2302755, 2368548, 2434341, 2500134, 2565927, 2631720, 2697513, 2763306, 2829099, 2894892, 2960685, 3026478, 3092271, 3158064, 3223857, 3289650, 3355443, 3421236, 3487029, 3552822, 3618615, 3684408, 3750201, 3815994, 3881787, 3947580, 4013373, 4079166, 4144959, 4210752, 4276545, 4342338, 4408131, 4473924, 4539717, 4605510, 4671303, 4737096, 4802889, 4868682, 4934475, 5000268, 5066061, 5131854, 5197647, 5263440, 5329233, 5395026, 5460819, 5526612, 5592405, 5658198, 5723991, 5789784, 5855577, 5921370, 5987163, 6052956, 6118749, 6184542, 6250335, 6316128, 6381921, 6447714, 6513507, 6579300, 6645093, 6710886, 6776679, 6842472, 6908265, 6974058, 7039851, 7105644, 7171437, 7237230, 7303023, 7368816, 7434609, 7500402, 7566195, 7631988, 7697781, 7763574, 7829367, 7895160, 7960953, 8026746, 8092539, 8158332, 8224125, 8289918, 8355711, 8421504, 8487297, 8553090, 8618883, 8684676, 8750469, 8816262, 8882055, 8947848, 9013641, 9079434, 9145227, 9211020, 9276813, 9342606, 9408399, 9474192, 9539985, 9605778, 9671571, 9737364, 9803157, 9868950, 9934743, 10000536, 10066329, 10132122, 10197915, 10263708, 10329501, 10395294, 10461087, 10526880, 10592673, 10658466, 10724259, 10790052, 10855845, 10921638, 10987431, 11053224, 11119017, 11184810, 11250603, 11316396, 11382189, 11447982, 11513775, 11579568, 11645361, 11711154, 11776947, 11842740, 11908533, 11974326, 12040119, 12105912, 12171705, 12237498, 12303291, 12369084, 12434877, 12500670, 12566463, 12632256, 12698049, 12763842, 12829635, 12895428, 12961221, 13027014, 13092807, 13158600, 13224393, 13290186, 13355979, 13421772, 13487565, 13553358, 13619151, 13684944, 13750737, 13816530, 13882323, 13948116, 14013909, 14079702, 14145495, 14211288, 14277081, 14342874, 14408667, 14474460, 14540253, 14606046, 14671839, 14737632, 14803425, 14869218, 14935011, 15000804, 15066597, 15132390, 15198183, 15263976, 15329769, 15395562, 15461355, 15527148, 15592941, 15658734, 15724527, 15790320, 15856113, 15921906, 15987699, 16053492, 16119285, 16185078, 16250871, 16316664, 16382457, 16448250, 16514043, 16579836, 16645629, 16711422] ("Array")
        w170 = u32 4417888
        n61 = local read "Trace Topography Array"() -> (w172:i32[][])
        "Trace  Topography" <- w172
        n62 = local read "Topography Array"() -> (→"Topography Image":i32[][])
        n63 = local read "Trace AI2 array"() -> (w173:i16[][])
        "Trace Frequency" <- w173
        n64 = local read "AI2 Array"() -> (→"Frequency Shift Image":i16[][])
        n65 = Array Max & Min(array=w173) -> (max value=w176:i16, min value=w175:i16)  [unwired: 2 out]
        n66 = property on="Frequency Shift Image" class="IntGraph (strict)"("ZScale.Maximum"=w176, "ZScale.Minimum"=w175) -> ()  [unwired: 2 in, 2 out]
        n67 = Array Max & Min(array=w172) -> (max value=w156:i32, min value=w159:i32)  [unwired: 2 out]
        n68 = property on="Topography Image" class="IntGraph (strict)"("ZScale.Maximum"=w156, "ZScale.Minimum"=w159) -> ()  [unwired: 2 in, 2 out]
        n69 = Greater?(x=w156, y=w155) -> (0:w158:bool)
        n70 = local read "Trace AI0 Array"() -> (w171:i16[][])
        "Trace Bottom Sensor Phase" <- w171
        n71 = Select(t=w156, s=w158, f=w155) -> (s? t:f=w157:i32)
        n72 = Array Max & Min(array=w171) -> (max value=w179:i16, min value=w178:i16)  [unwired: 2 out]
        n73 = local read "AI0 Array"() -> (→"Bottom Sensor Phase  Image":i16[][])
        n74 = property on="Topography Image" class="IntGraph (strict)"("Color Table"=w169, "ZScale.Low Color"=w170) -> ()  [unwired: 2 in, 2 out]
        n75 = property on="Bottom Sensor Phase  Image" class="IntGraph (strict)"("ZScale.Maximum"=w179, "ZScale.Minimum"=w178) -> ()  [unwired: 2 in, 2 out]
        n76 = property on="Bottom Sensor Phase  Image" class="IntGraph (strict)"("Color Table"=w169, "ZScale.Low Color"=w170) -> ()  [unwired: 2 in, 2 out]
        n77 = local read "Trace AI6  array"() -> (w166:i16[][])
        "Trace TF Magnitud" <- w166
        n78 = local read "AI6 Array"() -> (→"TF Magnitude Image":i16[][])
        n79 = Array Max & Min(array=w166) -> (max value=w165:i16, min value=w164:i16)  [unwired: 2 out]
        n80 = property on="Frequency Shift Image" class="IntGraph (strict)"("Color Table"=w169, "ZScale.Low Color"=w170) -> ()  [unwired: 2 in, 2 out]
        n81 = property on="TF Magnitude Image" class="IntGraph (strict)"("ZScale.Maximum"=w165, "ZScale.Minimum"=w164) -> ()  [unwired: 2 in, 2 out]
        n82 = local read "Trace AI5 array"() -> (w162:i16[][])
        "Trace Bottom Sensor Magnitude" <- w162
        n83 = local read "AI5 Array"() -> (→"Bottom Sensor Magnitude Image":i16[][])
        n84 = Array Max & Min(array=w162) -> (max value=w161:i16, min value=w160:i16)  [unwired: 2 out]
        n85 = property on="Bottom Sensor Magnitude Image" class="IntGraph (strict)"("ZScale.Maximum"=w161, "ZScale.Minimum"=w160) -> ()  [unwired: 2 in, 2 out]
      }
    }
  }
  n86 = Generate Occurrence() -> (w23:refnum<k4>)
  n87 = xnode "Close FPGA VI Reference"("FPGA VI Reference In"=w31, "error in"=w30) -> ("error out"=→"error out":errorcluster)
  n88 = while {
    tunnel: w23 -> [w180]
    stop <- FALSE stop-if-true
    n89 = case shown="False" "New Image" {
      tunnel: w180 -> [_ w183]
      frame False {
      }
      frame True {
        n90 = Set Occurrence(w183) -> ()
      }
    }
  }
  n91 = xnode "Open FPGA VI Reference"() -> ("FPGA VI Reference Out"=w32:refnum<k20>, "error out"=w26:errorcluster)  [unwired: 2 in]
  n92 = while {
    tunnel: w32 -> [w218]
    tunnel: [w219] -> w29
    tunnel: w26 -> [w217]
    tunnel: [w208] -> w25
    tunnel: w24 -> [w206]
    tunnel: w23 -> [w205]
    shift-right: [w199] -> _
    shift-left: TRUE -> [w195]
    shift-right: [w187] -> _
    shift-left: -1 ("image indicator") -> [w189]
    stop <- FALSE stop-if-true
    n93 = flat-sequence {
      tunnel: [w288] -> w216
      tunnel: [w279] -> w215
      tunnel: [w271] -> w214
      tunnel: [w277] -> w213
      tunnel: [w274] -> w212
      tunnel: [w242] -> w211
      tunnel: [w275] -> w210
      tunnel: [w287] -> w209
      tunnel: [w286] -> w207
      tunnel: w218 -> [w272]
      tunnel: w217 -> [w273]
      tunnel: w206 -> [w286]
      tunnel: [w270] -> w196
      tunnel: w195 -> [w264]
      tunnel: [w239] -> w192
      tunnel: [w247] -> w191
      tunnel: [w245] -> w190
      tunnel: w189 -> [w223]
      tunnel: [w230] -> w188
      tunnel: w216 -> [w318]
      tunnel: w215 -> [w317]
      tunnel: w214 -> [w304]
      tunnel: w213 -> [w316]
      tunnel: w212 -> [w314]
      tunnel: w211 -> [w306]
      tunnel: w210 -> [w312]
      tunnel: w209 -> [w315]
      tunnel: [w318] -> w204
      tunnel: [w315] -> w202
      tunnel: w207 -> [w309]
      tunnel: [w309] -> w200
      tunnel: [w308] -> w197
      tunnel: w196 -> [w308]
      tunnel: [w307] -> w193
      tunnel: w192 -> [w307]
      tunnel: w191 -> [w305]
      tunnel: w190 -> [w303]
      tunnel: w188 -> [w302]
      tunnel: [w302] -> w185
      tunnel: w204 -> [w379]
      tunnel: [w379] -> w203
      tunnel: w202 -> [w378]
      tunnel: [w378] -> w201
      tunnel: w200 -> [w374]
      tunnel: [w377] -> w198
      tunnel: w197 -> [w377]
      tunnel: [w376] -> w194
      tunnel: w193 -> [w376]
      tunnel: [w375] -> w186
      tunnel: w185 -> [w375]
      tunnel: [w374] -> w184
      tunnel: [w385] -> w208
      tunnel: [w386] -> w219
      tunnel: w203 -> [w386]
      tunnel: w201 -> [w385]
      tunnel: w205 -> [w384]
      tunnel: [w383] -> w199
      tunnel: w198 -> [w383]
      tunnel: w194 -> [w382]
      tunnel: [w381] -> w187
      tunnel: w186 -> [w381]
      tunnel: w184 -> [w380]
      frame #0 {
        # "1024 is just a number\nlarger than 512 but less\nthan total pixel images"
        n94 = local read "X axis pixels"() -> (w261:u16)
        n95 = xnode "Invoke Method"("FPGA VI Reference In"=w272, "error in"=w273, "Number of Elements"=w261, "Timeout (ms)"=-1) -> ("FPGA VI Reference Out"=w285:refnum<k20>, "error out"=w284:errorcluster, "Data"=w260:u64[])  [unwired: 1 out]
        n96 = Decimate 1D Array(w260) -> (w259:u64[], w256:u64[])
        n97 = local read "Pixels for one image"() -> (w267:i32)
        n98 = To Unsigned Long Integer(number=w256) -> (unsigned 32bit integer=w255:u32[])
        n99 = Split Number(x=w259) -> (hi(x)=w297:u32[], lo(x)=w296:u32[])
        n100 = Split Number(x=w255) -> (hi(x)=w252:u16[], lo(x)=w249:u16[])
        n101 = xnode "Read/Write Control"("FPGA VI Reference In"=w285, "error in"=w284) -> ("FPGA VI Reference Out"=w282:refnum<k20>, "error out"=w283:errorcluster, "Indicator  forth/back X axis"=w242:i8, "iterations x"=w266:i32, "Y line"=w227:i32)
        "Y line" <- w227
        n102 = Less Or Equal?(x=w266, y=w261) -> (x <= y?=w265:bool)
        n103 = Split Number(x=w297) -> (hi(x)=w295:u16[], lo(x)=w229:u16[])
        "hi(x)" <- w229
        n104 = Split Number(x=w296) -> (hi(x)=w292:u16[], lo(x)=w290:u16[])
        n105 = local read "Y axis pixels"() -> (w226:u16)
        n106 = Select(t=TRUE, s=w265, f=w264) -> (s? t:f=w263:bool)
        n107 = First Call?() -> (First Call?: T/F=w228:bool)
        n108 = Increment(x=w266) -> (x+1=w269:i32)
        n109 = xnode "Invoke Method"("FPGA VI Reference In"=w282, "error in"=w283, "Number of Elements"=w261, "Timeout (ms)"=-1) -> ("FPGA VI Reference Out"=w288:refnum<k20>, "error out"=w287:errorcluster, "Data"=w258:u64[])  [unwired: 1 out]
        n110 = Quotient & Remainder(x=w269, y=w267) -> (x-y*floor(x/y)=w237:i32)  [unwired: 1 out]
        n111 = Less Or Equal?(x=w237, y=w261) -> (x <= y?=w234:bool)
        n112 = Decrement(x=w226) -> (x-1=w221:u16)
        n113 = Quotient & Remainder(x=w227, y=w221) -> (floor(x/y)=w225:i32)  [unwired: 1 out]
        "fpga y images" <- w225
        n114 = Add(x=w225, y=w223) -> (x+y=w224:i32)
        n115 = Select(t=w224, s=w228, f=w223) -> (s? t:f=w222:i32)
        n116 = Increment(x=w222) -> (x+1=w233:i32)
        n117 = Select(t=w233, s=w234, f=w222) -> (s? t:f=w230:i32)
        "line shift" <- w230
        n118 = Increment(x=w230) -> (x+1=→"image indicator":i32)
        n119 = Add(x=w227, y=w230) -> (x+y=w231:i32)
        n120 = Quotient & Remainder(x=w231, y=w226) -> (x-y*floor(x/y)=w238:i32)  [unwired: 1 out]
        n121 = Decimate 1D Array(w258) -> (w257:u64[], w254:u64[])
        n122 = Not(x=w263) -> (.not. x?=w268:bool)
        n123 = To Unsigned Long Integer(number=w254) -> (unsigned 32bit integer=w253:u32[])
        n124 = Select(t=w268, s=w234, f=w263) -> (s? t:f=w270:bool)
        n125 = Split Number(x=w253) -> (hi(x)=w251:u16[], lo(x)=w250:u16[])
        n126 = Split Number(x=w257) -> (hi(x)=w301:u32[], lo(x)=w300:u32[])
        n127 = Split Number(x=w301) -> (hi(x)=w294:u16[], lo(x)=w293:u16[])
        n128 = Split Number(x=w300) -> (hi(x)=w291:u16[], lo(x)=w289:u16[])
        n129 = Equal?(x=w242, y=i8 -1) -> (x = y?=w240:bool)
        n130 = Subtract(x=w221, y=w238) -> (x-y=w281:i32)
        n131 = Equal?(x=w238, y=255) -> (x = y?=w244:bool)
        n132 = Greater?(x=w237, y=1024) -> (0:w235:bool)
        n133 = Select(t=w238, s=w270, f=w281) -> (s? t:f=w271:i32)
        "line in matrix" <- w271
        n134 = Compound Arithmetic op=AND(w235, w244, w240) -> (w239:bool)
        n135 = Build Array (concatenate)(w252, w251) -> (w248:u16[])
        n136 = Build Array (concatenate)(w249, w250) -> (w246:u16[])
        n137 = Build Array (concatenate)(w292, w291) -> (w274:u16[])
        n138 = Build Array (concatenate)(w290, w289) -> (w276:u16[])
        n139 = Build Array (concatenate)(w229, w293) -> (w278:u16[])
        n140 = Build Array (concatenate)(w295, w294) -> (w280:u16[])
        n141 = To Word Integer(number=w248) -> (16bit integer=w247:i16[])
        n142 = To Word Integer(number=w246) -> (16bit integer=w245:i16[])
        n143 = To Word Integer(number=w278) -> (16bit integer=w277:i16[])
        n144 = To Word Integer(number=w280) -> (16bit integer=w279:i16[])
        n145 = To Word Integer(number=w276) -> (16bit integer=w275:i16[])
      }
      frame #1 {
        n146 = Multiply(x=w314, y=65535) -> (x*y=w311:i32[])
        n147 = Add(x=w311, y=w312) -> (x+y=w310:i32[])
        n148 = case shown="-1" w306 {
          tunnel: w310 -> [w341 w351]
          tunnel: w304 -> [w343 w348]
          frame 1, Default {
            n149 = local read "Topography Array"() -> (w344:i32[][])
            n150 = Replace Array Subset(array=w344, new element=w341, index (col)=w343) -> (w342:i32[][])  [unwired: 1 in]
            n151 = local write "Topography Array"(w342) -> ()
            "Trace Topography Array temp" <- w341
          }
          frame -1 {
            n152 = local read "Trace Topography Array temp"() -> (w345:i32[])
            n153 = Reverse 1D Array(array=w351) -> (reversed array=w347:i32[])
            n154 = local read "Topography Array back"() -> (w349:i32[][])
            n155 = Build Array(w345, w347) -> (→"Trace Topography Array":i32[][])
            n156 = Replace Array Subset "Replace Array Subset"(array=w349, new element=w347, index (col)=w348) -> (w350:i32[][])  [unwired: 1 in]
            n157 = local write "Topography Array back"(w350) -> ()
          }
        }
        n158 = case shown="-1" w306 {
          tunnel: w305 -> [w336 w340]
          tunnel: w304 -> [w335 w338]
          frame -1 {
            n159 = local read "AI6 Array Back"() -> (w334:i16[][])
            n160 = Reverse 1D Array(array=w336) -> (reversed array=w331:i16[])
            n161 = local read "TraceAI6 temp"() -> (w332:i16[])
            n162 = Replace Array Subset(array=w334, new element=w331, index (col)=w335) -> (w333:i16[][])  [unwired: 1 in]
            n163 = local write "AI6 Array Back"(w333) -> ()
            n164 = Build Array(w332, w331) -> (→"Trace AI6  array":i16[][])
          }
          frame 1, Default {
            n165 = local read "AI6 Array"() -> (w339:i16[][])
            n166 = Replace Array Subset(array=w339, new element=w340, index (col)=w338) -> (w337:i16[][])  [unwired: 1 in]
            n167 = local write "AI6 Array"(w337) -> ()
            "TraceAI6 temp" <- w340
          }
        }
        n168 = case shown="-1" w306 {
          tunnel: w316 -> [w352 w362]
          tunnel: w304 -> [w353 w359]
          frame 1, Default {
            n169 = local read "AI2 Array"() -> (w355:i16[][])
            n170 = Replace Array Subset(array=w355, new element=w352, index (col)=w353) -> (w354:i16[][])  [unwired: 1 in]
            n171 = local write "AI2 Array"(w354) -> ()
            "TraceAI2 array temp" <- w352
          }
          frame -1 {
            n172 = local read "TraceAI2 array temp"() -> (w356:i16[])
            n173 = Reverse 1D Array(array=w362) -> (reversed array=w357:i16[])
            n174 = local read "AI2 Array back"() -> (w361:i16[][])
            n175 = Replace Array Subset(array=w361, new element=w357, index (col)=w359) -> (w360:i16[][])  [unwired: 1 in]
            n176 = Build Array(w356, w357) -> (→"Trace AI2 array":i16[][])
            n177 = local write "AI2 Array back"(w360) -> ()
          }
        }
        n178 = case shown="-1" w306 {
          tunnel: w317 -> [w363 w373]
          tunnel: w304 -> [w366 w370]
          frame 1, Default {
            n179 = local read "AI0 Array"() -> (w365:i16[][])
            n180 = Replace Array Subset(array=w365, new element=w363, index (col)=w366) -> (w364:i16[][])  [unwired: 1 in]
            n181 = local write "AI0 Array"(w364) -> ()
            "Trace AI0 array temp" <- w363
          }
          frame -1 {
            n182 = local read "Trace AI0 array temp"() -> (w369:i16[])
            n183 = Reverse 1D Array(array=w373) -> (reversed array=w368:i16[])
            n184 = local read "AI0 back"() -> (w372:i16[][])
            n185 = Replace Array Subset(array=w372, new element=w368, index (col)=w370) -> (w371:i16[][])  [unwired: 1 in]
            n186 = Build Array(w369, w368) -> (→"Trace AI0 Array":i16[][])
            n187 = local write "AI0 back"(w371) -> ()
          }
        }
        n188 = case shown="-1" w306 {
          tunnel: w304 -> [w323 w329]
          tunnel: w303 -> [w325 w326]
          frame -1 {
            n189 = local read "AI5 Back"() -> (w324:i16[][])
            n190 = Reverse 1D Array(array=w325) -> (reversed array=w321:i16[])
            n191 = local read "Trace AI5 temp"() -> (w320:i16[])
            n192 = Replace Array Subset(array=w324, new element=w321, index (col)=w323) -> (w322:i16[][])  [unwired: 1 in]
            n193 = local write "AI5 Back"(w322) -> ()
            n194 = Build Array(w320, w321) -> (→"Trace AI5 array":i16[][])
          }
          frame 1, Default {
            n195 = local read "AI5 Array"() -> (w328:i16[][])
            n196 = Replace Array Subset(array=w328, new element=w326, index (col)=w329) -> (w327:i16[][])  [unwired: 1 in]
            n197 = local write "AI5 Array"(w327) -> ()
            "Trace AI5 temp" <- w326
          }
        }
      }
      frame #2 {
        n198 = Set Occurrence(w374) -> ()
      }
      frame #3 {
        n199 = case shown="True" w382 {
          tunnel: w384 -> [_ w389]
          tunnel: w380 -> [_ w388]
          frame False {
          }
          frame True {
            n200 = flat-sequence {
              tunnel: w389 -> [w391]
              tunnel: w388 -> [w390]
              tunnel: [w390] -> w387
              tunnel: w387 -> [w392]
              frame #0 {
                n201 = Set Occurrence(w391) -> ()
              }
              frame #1 {
                n202 = while {
                  tunnel: w392 -> [w393]
                  stop <- w394 continue-if-true
                  n203 = Wait on Occurrence(2:w393) -> (0:w394:bool)  [unwired: 2 in]
                }
              }
            }
          }
        }
      }
    }
  }
  n204 = while {
    tunnel: w23 -> [w399]
    tunnel: w24 -> [w395]
    stop <- FALSE stop-if-true
    n205 = flat-sequence {
      tunnel: [w409] -> w398
      tunnel: w399 -> [w409]
      tunnel: [w408] -> w396
      tunnel: w395 -> [w408]
      tunnel: w398 -> [w414]
      tunnel: [w414] -> w397
      tunnel: w396 -> [w413]
      tunnel: w397 -> [w415]
      frame #0 {
        w401 = i16 0 ("element")
        w407 = i16 0 ("element")
        n206 = local read "Y axis pixels"() -> (w405:u16)
        n207 = local read "X axis pixels"() -> (w406:u16)
        n208 = Initialize Array(0 ("element"), w405, w406) -> (→"Topography Array" →"Topography Array back":i32[][])
        n209 = Initialize Array(w401, w405, w406) -> (→"AI6 Array" →"AI6 Array Back":i16[][])
        n210 = Initialize Array(w401, w405, w406) -> (→"AI0 Array" →"AI0 back":i16[][])
        n211 = Initialize Array(w407, w405, w406) -> (→"AI2 Array" →"AI2 Array back":i16[][])
        n212 = Initialize Array(w407, w405, w406) -> (→"AI5 Array" →"AI5 Back":i16[][])
      }
      frame #1 {
        n213 = Set Occurrence(w413) -> ()
      }
      frame #2 {
        n214 = while {
          tunnel: w415 -> [w416]
          stop <- w417 continue-if-true
          n215 = Wait on Occurrence(2:w416) -> (0:w417:bool)  [unwired: 2 in]
        }
      }
      frame #3 {
        w424 = TRUE ("transpose? (no:F)")
        w425 = "," ("delimiter (\\t)")
        w432 = ".csv" ("string")
        w433 = "-rev" ("string")
        w430 = "%.6f" ("format (%.3f)")
        w442 = ".csv" ("string")
        w456 = "%.6f" ("format (%.3f)")
        n216 = Get Date/Time In Seconds() -> (seconds since 1Jan1904=w482:timestamp)
        n217 = Format Date/Time String(time format string (%c)="%Y-%m-%d-%H-%M-%S", seconds (now)=w482) -> (date/time string=w419:string)  [unwired: 1 in]
        n218 = Concatenate Strings(w419, "Freq Prefix 1", "Freq Prefix 2", "AI2" ("string")) -> (w445:string)
        n219 = Concatenate Strings(w445, ".csv" ("string")) -> (w479:string)
        n220 = Concatenate Strings(w419, "Phase Prefix 1", "Phase Prefix 2", "AI0" ("string")) -> (w447:string)
        n221 = Concatenate Strings(w419, "Topo Prefix 1", "Topo Prefix 2", "Topography" ("string")) -> (w451:string)
        n222 = Concatenate Strings(w451, ".csv" ("string")) -> (w468:string)
        n223 = Concatenate Strings(w447, ".csv" ("string")) -> (w469:string)
        n224 = local read "AI5 Array"() -> (w429:i16[][])
        n225 = local read "AI6 Array"() -> (w428:i16[][])
        n226 = Build Path(base path="Data Directory", name or relative path=w469) -> (appended path=w467:path)
        n227 = Build Path(base path="Data Directory", name or relative path=w468) -> (appended path=w466:path)
        n228 = Build Path(base path="Data Directory", name or relative path=w479) -> (appended path=w478:path)
        n229 = local read "Topography Array"() -> (w465:i32[][])
        n230 = local read "AI0 Array"() -> (w464:i16[][])
        n231 = local read "AI2 Array"() -> (w485:i16[][])
        n232 = Concatenate Strings(w419, "AI6" ("string")) -> (w431:string)
        n233 = Concatenate Strings(w419, "AI5" ("string")) -> (w439:string)
        n234 = Concatenate Strings(w431, w442) -> (w441:string)
        n235 = Concatenate Strings(w439, w442) -> (w444:string)
        n236 = Build Path(base path="Data Directory", name or relative path=w444) -> (appended path=w443:path)
        n237 = call-poly <vilib>:"Write To Spreadsheet File.vi"("delimiter (\\t)"=w425, "transpose? (no:F)"=w424, "format (%d)"="%.6f" ("format (%.3f)"), "2D data"=w465, "file path (dialog if empty)"=w466) -> ()  [unwired: 3 in, 1 out]
        n238 = Build Path(base path="Data Directory", name or relative path=w441) -> (appended path=w440:path)
        n239 = call-poly <vilib>:"Write To Spreadsheet File.vi"("delimiter (\\t)"=w425, "transpose? (no:F)"=w424, "format (%d)"="%.6f" ("format (%.3f)"), "2D data"=w464, "file path (dialog if empty)"=w467) -> ()  [unwired: 3 in, 1 out]
        n240 = call-poly <vilib>:"Write To Spreadsheet File.vi"("delimiter (\\t)"=w425, "transpose? (no:F)"=w424, "format (%d)"=w456, "2D data"=w485, "file path (dialog if empty)"=w478) -> ()  [unwired: 3 in, 1 out]
        n241 = call-poly <vilib>:"Write To Spreadsheet File.vi"("delimiter (\\t)"=w425, "transpose? (no:F)"=w424, "format (%d)"=w430, "2D data"=w428, "file path (dialog if empty)"=w440) -> ()  [unwired: 3 in, 1 out]
        n242 = call-poly <vilib>:"Write To Spreadsheet File.vi"("delimiter (\\t)"=w425, "transpose? (no:F)"=w424, "format (%d)"=w430, "2D data"=w429, "file path (dialog if empty)"=w443) -> ()  [unwired: 3 in, 1 out]
        n243 = Concatenate Strings(w445, "-rev" ("string"), ".csv" ("string")) -> (w461:string)
        n244 = local read "AI2 Array back"() -> (w446:i16[][])
        n245 = Concatenate Strings(w447, "-rev" ("string"), ".csv" ("string")) -> (w449:string)
        n246 = Concatenate Strings(w451, "-rev" ("string"), ".csv" ("string")) -> (w452:string)
        n247 = local read "Topography Array back"() -> (w455:i32[][])
        n248 = local read "AI0 back"() -> (w454:i16[][])
        n249 = Build Path(base path="Data Directory", name or relative path=w449) -> (appended path=w448:path)
        n250 = Build Path(base path="Data Directory", name or relative path=w461) -> (appended path=w453:path)
        n251 = local read "AI5 Back"() -> (w427:i16[][])
        n252 = local read "AI6 Array Back"() -> (w426:i16[][])
        n253 = Build Path(base path="Data Directory", name or relative path=w452) -> (appended path=w450:path)
        n254 = call-poly <vilib>:"Write To Spreadsheet File.vi"("delimiter (\\t)"=w425, "transpose? (no:F)"=w424, "format (%d)"=w456, "2D data"=w446, "file path (dialog if empty)"=w453) -> ()  [unwired: 3 in, 1 out]
        n255 = call-poly <vilib>:"Write To Spreadsheet File.vi"("delimiter (\\t)"=w425, "transpose? (no:F)"=w424, "format (%d)"=w456, "2D data"=w454, "file path (dialog if empty)"=w448) -> ()  [unwired: 3 in, 1 out]
        n256 = call-poly <vilib>:"Write To Spreadsheet File.vi"("delimiter (\\t)"=w425, "transpose? (no:F)"=w424, "format (%d)"=w456, "2D data"=w455, "file path (dialog if empty)"=w450) -> ()  [unwired: 3 in, 1 out]
        n257 = Concatenate Strings(w439, w433, w432) -> (w438:string)
        n258 = Concatenate Strings(w431, w433, w432) -> (w435:string)
        n259 = Build Path(base path="Data Directory", name or relative path=w438) -> (appended path=w437:path)
        n260 = Build Path(base path="Data Directory", name or relative path=w435) -> (appended path=w436:path)
        n261 = call-poly <vilib>:"Write To Spreadsheet File.vi"("delimiter (\\t)"=w425, "transpose? (no:F)"=w424, "format (%d)"=w430, "2D data"=w426, "file path (dialog if empty)"=w436) -> ()  [unwired: 3 in, 1 out]
        n262 = call-poly <vilib>:"Write To Spreadsheet File.vi"("delimiter (\\t)"=w425, "transpose? (no:F)"=w424, "format (%d)"=w430, "2D data"=w427, "file path (dialog if empty)"=w437) -> ()  [unwired: 3 in, 1 out]
      }
    }
  }
  n263 = xnode "Close FPGA VI Reference"("FPGA VI Reference In"=w29, "error in"=w25) -> ("error out"=→"error out 2":errorcluster)
